vi "Taher.vi"() -> ()   [LabVIEW 2017]
doc: "I. Description:\nThis example demonstrates how to continuously acquire and generate data at the same time, synchronized with one another.\n\nII. Instructions for Running:\n1. Select the physical channel to correspond to where your signal is input on the DAQ device. Also, select the corresponding channel for where your signal is being generated.\n2. Enter the minimum and maximum voltage ranges.\nNote: For better accuracy try to match the input range to the expected voltage level of the measured signal.\n3. Set the sample rate of the acquisition.\nNote: The rate should be at least twice as fast as the maximum frequency component of the signal being acquired. \n6. Select the Rate for the generation\n7. Select what type of signal to generate and the amplitude.\nNote: This example requires two DMA channels to run. If your hardware does not support two DMA channels, you need to set the Data Transfer Mechanism property for the Analog Output Task to use \"Interrupts\". The Data Transfer Mechanism property is located in the DAQmx Channel Property hierarchy at:\n\nDAQmx Channel Property Node>>Analog Output>>General Properties>>Advanced>>Data Transfer and Memory>>Data Transfer Mechanism\n\nRefer to your device documentation to determine how many DMA channels are supported for your hardware.\n\nIII. Block Diagram Steps:\n1. Create an analog input voltage channel. Also, create an analog output voltage channel.\n2. Set the rate for the sample clock. Additionally, define the sample mode to be continuous. Also, set the sample clock rate for the signal generation.\n2a. Call the Get Terminal Name with Device Prefix VI. This will take a Task and a terminal and create a properly formatted device + terminal name to use as the source of the Trigger.\n3. Define the parameters for a Digital Edge Start Trigger. Set the Analog output to trigger off the AI Start Trigger. This is an internal trigger signal.\n4. Use the Basic Function Generator VI to create the signal to be generated.\n5. Call the Start VI to arm the two functions. Make sure the analog output is armed before the analog input. This will ensure both will start at the same time.\n6. Read the waveform data in a loop until the user hits the stop button or an error occurs. The Is Task Done? VI is used to check for errors in the Analog Output Task.\n7. Call the Clear VI to Clear the Task\n8. Use the popup dialog box to display an error if any.\n\nIV. I/O Connections Overview:\nMake sure your signal input/output terminals match the Physical Channel I/O controls."
uses:
  <vilib>/Utility/error.llb/DialogType.ctl
  <vilib>/DAQmx/configure/timing.llb/DAQmx Timing (Sample Clock).vi
  <vilib>/DAQmx/create/channels.llb/DAQmx Create Channel (AI-Voltage-Basic).vi
  <vilib>/DAQmx/create/channels.llb/DAQmx Create Channel (AO-Voltage-Basic).vi
  <vilib>/DAQmx/read.llb/DAQmx Read (Analog 1D DBL NChan 1Samp).vi
  <vilib>/DAQmx/write.llb/DAQmx Write (Analog DBL 1Chan 1Samp).vi
  <vilib>/Utility/file.llb/Write To Spreadsheet File (DBL).vi
  <vilib>/DAQmx/write.llb/DAQmx Write (Analog 2D DBL NChan NSamp).vi
  <vilib>/DAQmx/configure/trigger.llb/DAQmx Start Trigger (Digital Edge).vi
  <vilib>/DAQmx/read.llb/DAQmx Read (Analog DBL 1Chan 1Samp).vi
  pid/pid.llb/PID (DBL).vi
  pid/pid.llb/PID Output Rate Limiter (DBL).vi
  <vilib>/DAQmx/write.llb/DAQmx Write (Analog 1D DBL NChan 1Samp).vi
  <vilib>/ptbypt/NI_PtbyPt.lvlib
  <resource>/objmgr/daqmx.rc
  <vilib>/Analysis/NI_AALBase.lvlib
  <vilib>/Analysis/baseanly.llb/Mean (DBL).vi
  <vilib>/Analysis/NI_AALPro.lvlib
  <vilib>/Utility/file.llb/Write To Spreadsheet File (string).vi
panel:
  in  "Current Amplifier\n1/Gain  (A/V)":dbl=1.0 format="%#_13g"
  out "date/time string":string
  out "Bias Sweep 2":dbl[](graph)
  out "Array":dbl[](array[numeric])
  out "intercept":dbl
  out "Resistance \n[AI1 must be Vout]":dbl
  out "RTD-IV":cluster{dbl[], dbl[]}(graph)
  in  "Bias Offset Correct":dbl
  out "Bias Sweep":dbl[](graph)
  out "element":dbl
  out "mean":dbl format="%.6f"
  out "size(s)":i32
  out "Numeric":i32
  in  "PID":bool=TRUE caption="Step Z"
  in  "Tab Control":enum32{"PID Controller", "Tapping Controls"}(tab)=enum."Tapping Controls"
  in  "Proportional Gain":dbl=0.0001
  in  "Integral Gain":dbl=1e-07
  in  "Differential Gain":dbl=1e-05
  in  "Setpoint":dbl=0.1
  in  "Piezo Delta rate":dbl=1000.0
  in  "Min Current":dbl=0.002
  in  "Max Current":dbl=10.2
  in  "Ramp Rate":dbl=20.0
  in  "Make Contact":i32=1200
  in  "Break Contact":i32=500
  in  "Step Length":i32=100
  in  "Step Max":dbl=0.3
  in  "Step Min":dbl=0.05
  out "Tapping Stop":bool
  out "Case":i32
  in  "Contact Cycles":i32
  in  "Tapping":bool caption="Step Z"
  out "x/y":dbl
  out "Waveform Chart":dbl(graph)
  in  "Analog Ouyput 1":dbl(slide) min=-10.0 max=10.0 step=0.001 scale=-10.0..10.0
  in  "Manual Z":bool caption="Step Z"
  in  "Sweep Amplitude":dbl=1.0
  in  "Stop Sweep":bool
  out "Connections 2":string="AI0=Current\nAI1=Bias\nAI2=dI/dV\nAI3=d2I/dV2\nAI4=X-Axis\nAI5=Z-Axis\n"
  out "Connections":string="AO0=Bias\nAO1=Z-axis\nAO2=X-Axis\nAO3=NA"
  out "Save Indicator":bool
  in  "Z-Direction":bool caption="Step Z"
  in  "Update Bias":bool
  in  "Save IV":bool
  in  "Save Decay":bool
  in  "Sweep Bias":bool
  in  "Step Z":bool
  in  "Comments and Experimental Notes":string="Molecule=TP4\nGain=10nA\nBias Gain=div/1\nSweep Freq.=0.0008Hz\nRef. Bias=4mV\nRef. Freq=2.977kHz\nGain LIA1=2mV\nTC LIA1=1s\nGain LIA2=5mV\nTC LIA2=1s\nLIA1=EGG\nLIA2=SRS\nEGG is driving(possible 5mV offset)"
  in  "Filenumber":i32
  in  "DATA Filename":string="Data_"
  in  "Data Directory":path=path "E:/Research/Data"
  out "Current Decay":cluster{dbl[], dbl[]}(graph)
  out "d2I/dV2":cluster{dbl[], dbl[]}(graph)
  out "dI/dV":cluster{dbl[], dbl[]}(graph)
  out "IV":cluster{dbl[], dbl[]}(graph)
  in  "# Samples":i32=2000
  in  "Frequency (Hz)":dbl=1.0
  out "Measurement 2":cluster{i32, dbl, dbl[]}(graph) caption="Measurement"
  out "Actual Update Generation Rate 2":dbl=5000.0 caption="Actual Update Generation Rate" format="%0.2f"
  in  "stop 3":bool
  in  "Bias":dbl=0.1 caption="Bias Start Point" step=0.1 format="%_3g"
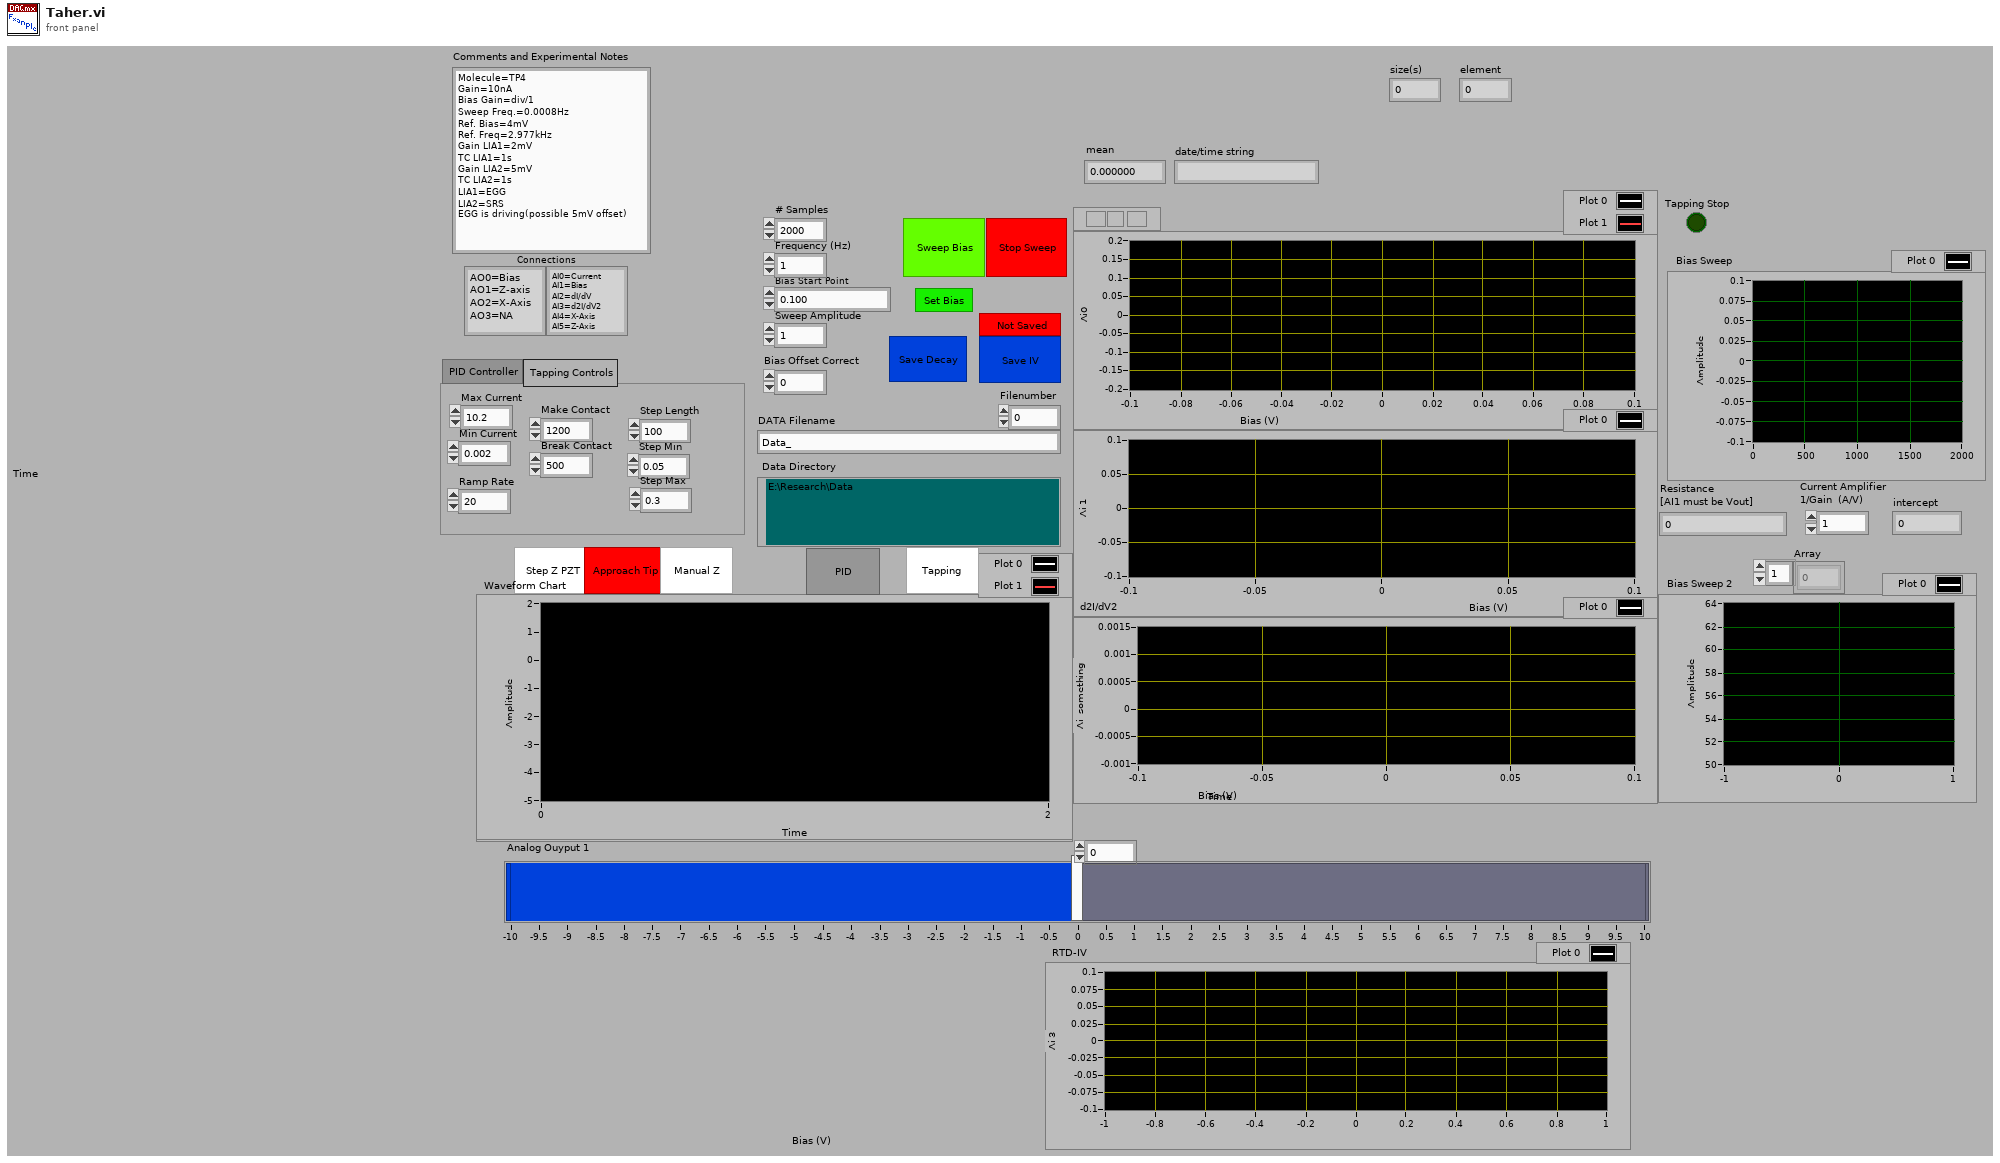
[diagram p1: front panel]
types:
  T1 = enum16{"open", "replace", "create", "open or create", "replace or create", "replace or create with confirmation"}
  T2 = typedef "DialogType.ctl" = u16
  T3 = cluster{"Proportional Gain":dbl, "Integral Gain ":dbl, "Differential Gain":dbl}
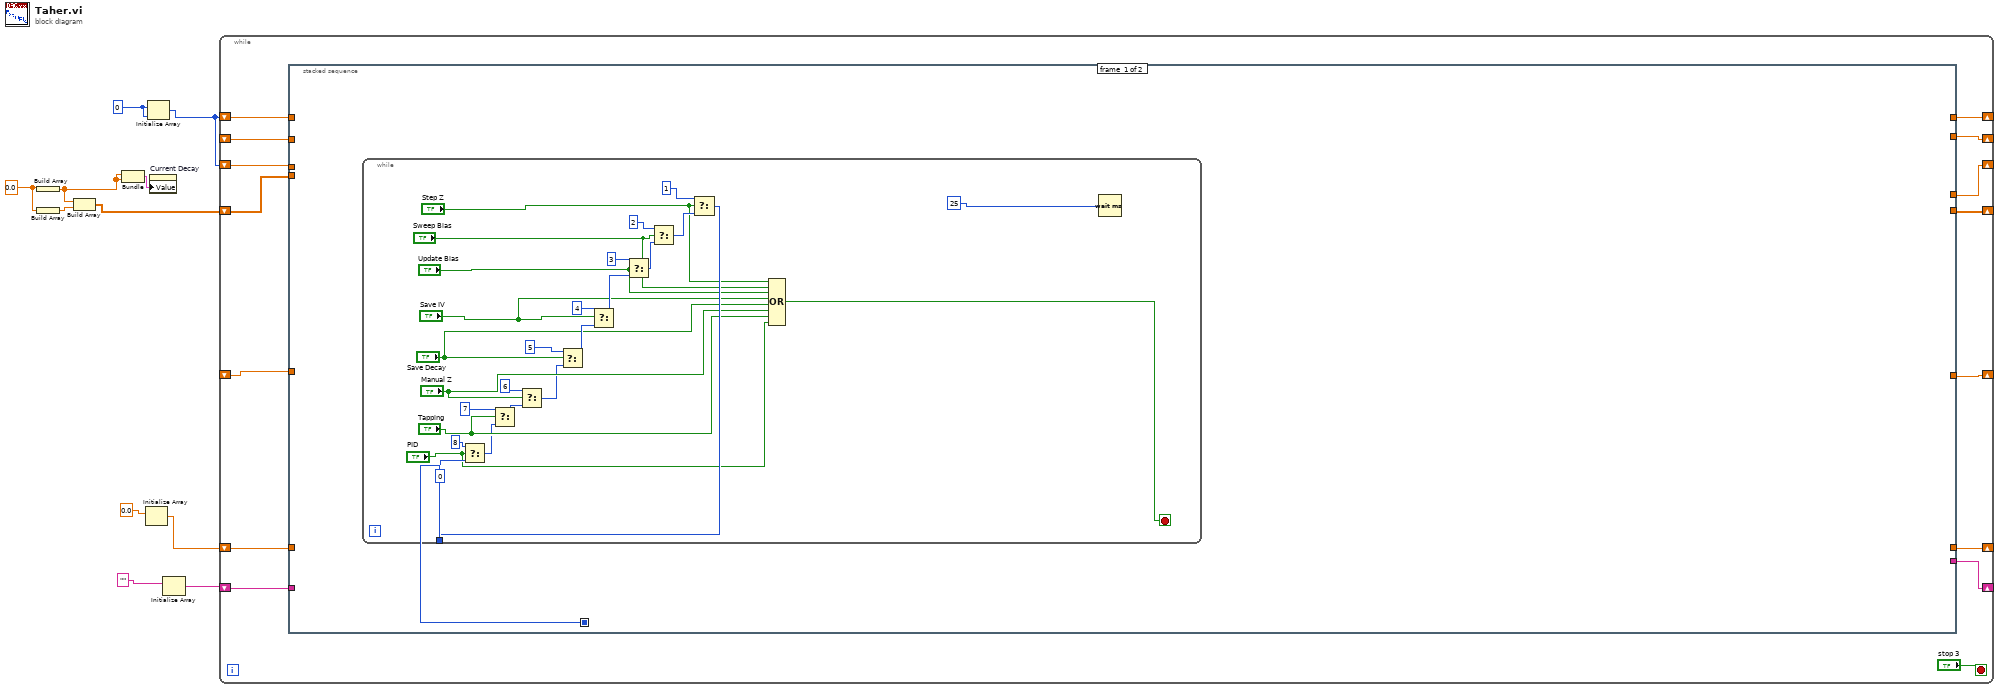
[diagram p0: block diagram]
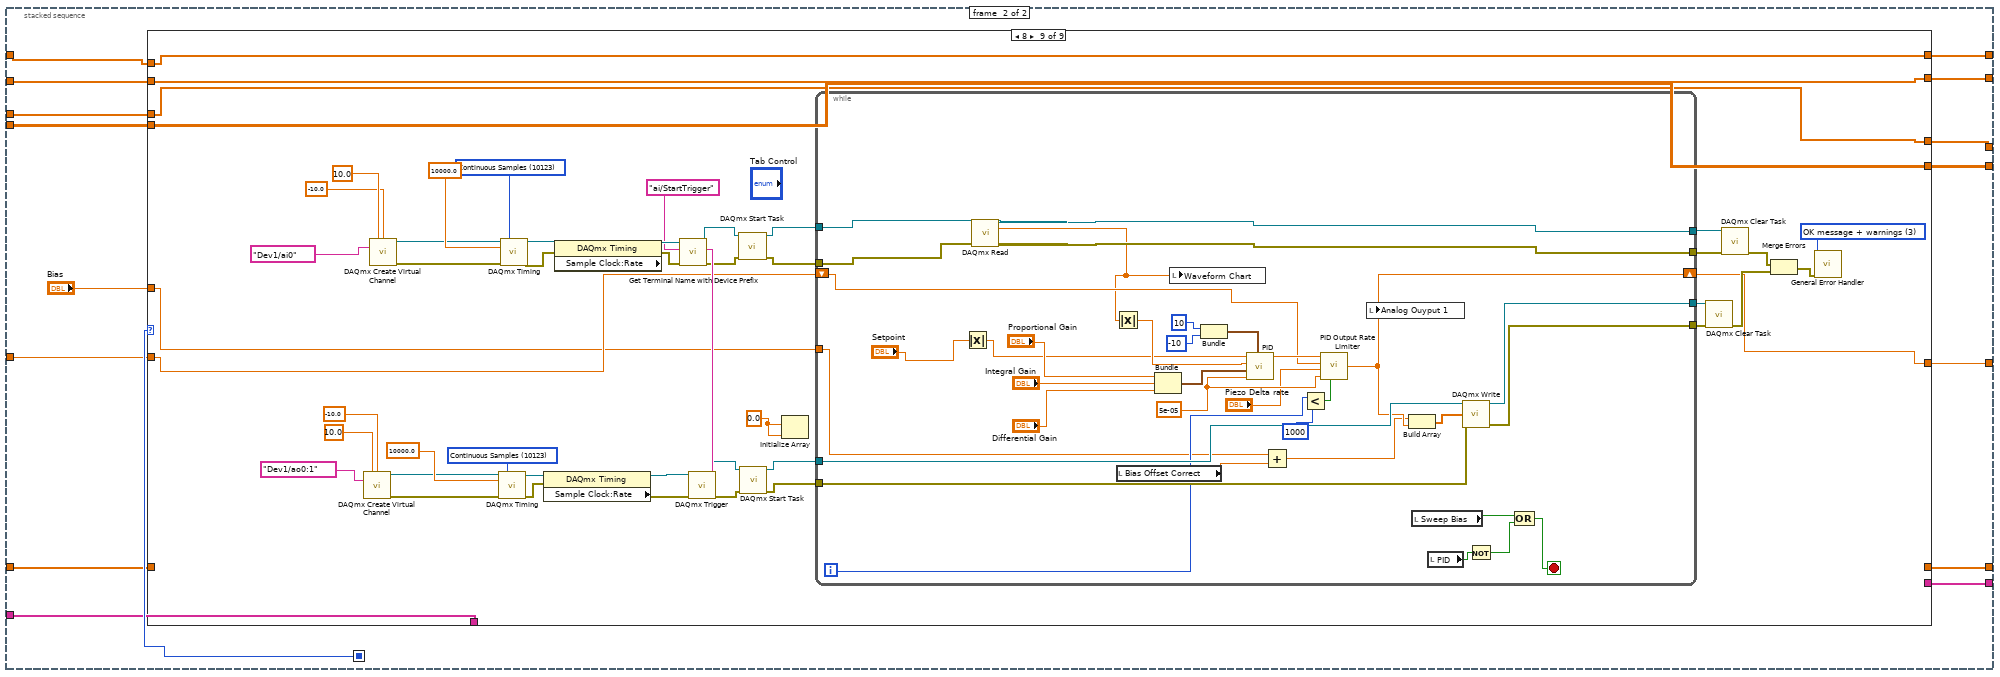
[diagram p2: hidden frame]
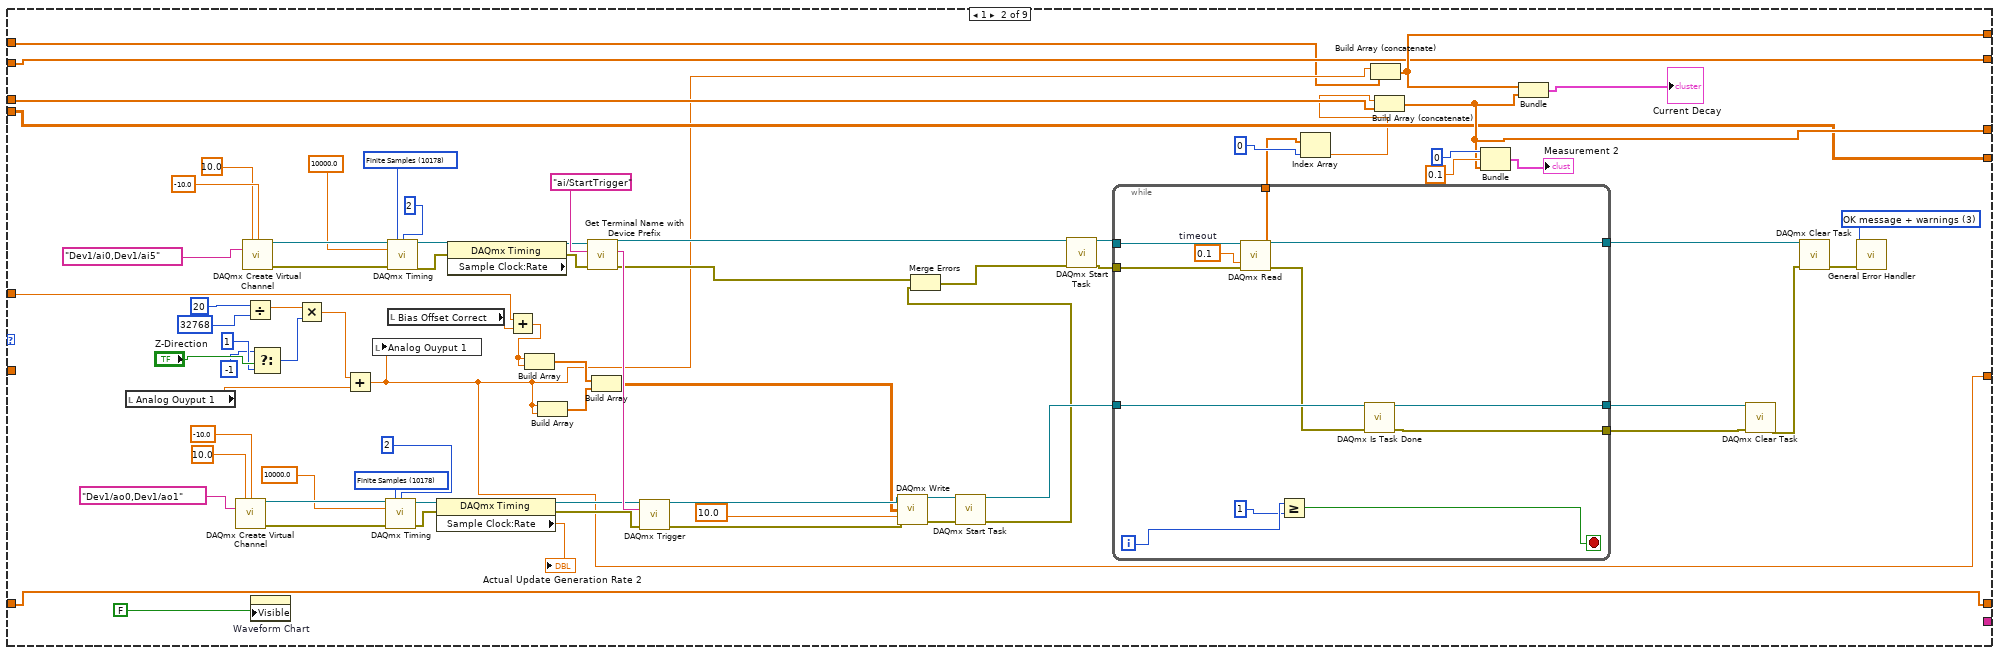
[diagram p4: hidden frame]
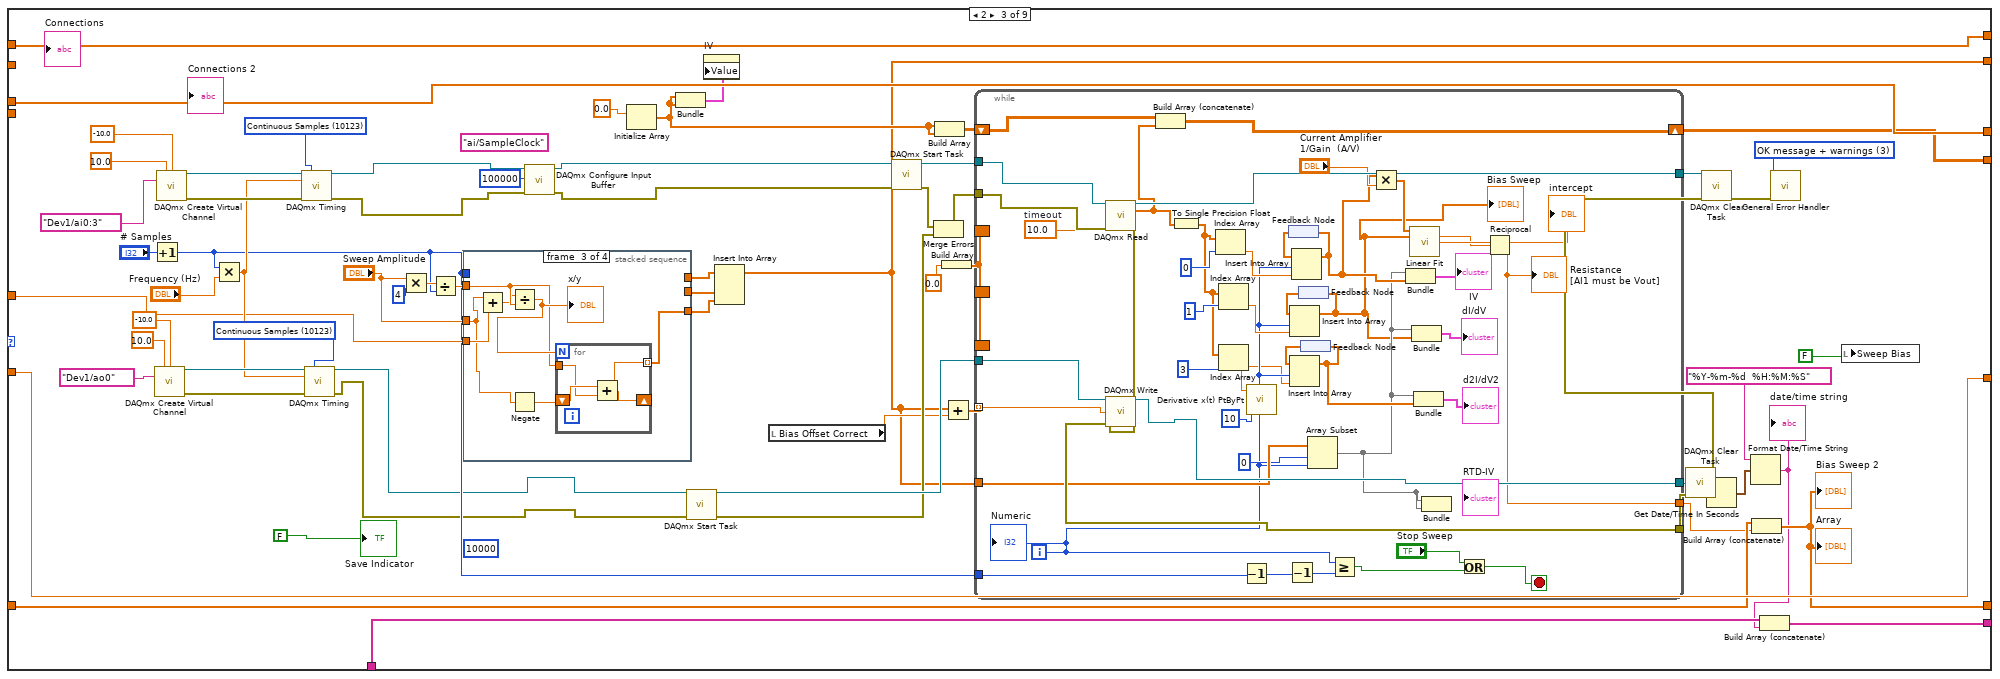
[diagram p5: hidden frame]
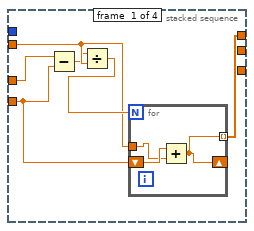
[diagram p6: hidden frame]
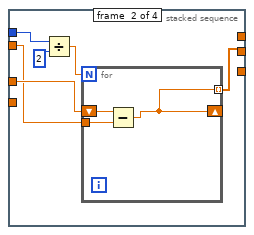
[diagram p7: hidden frame]
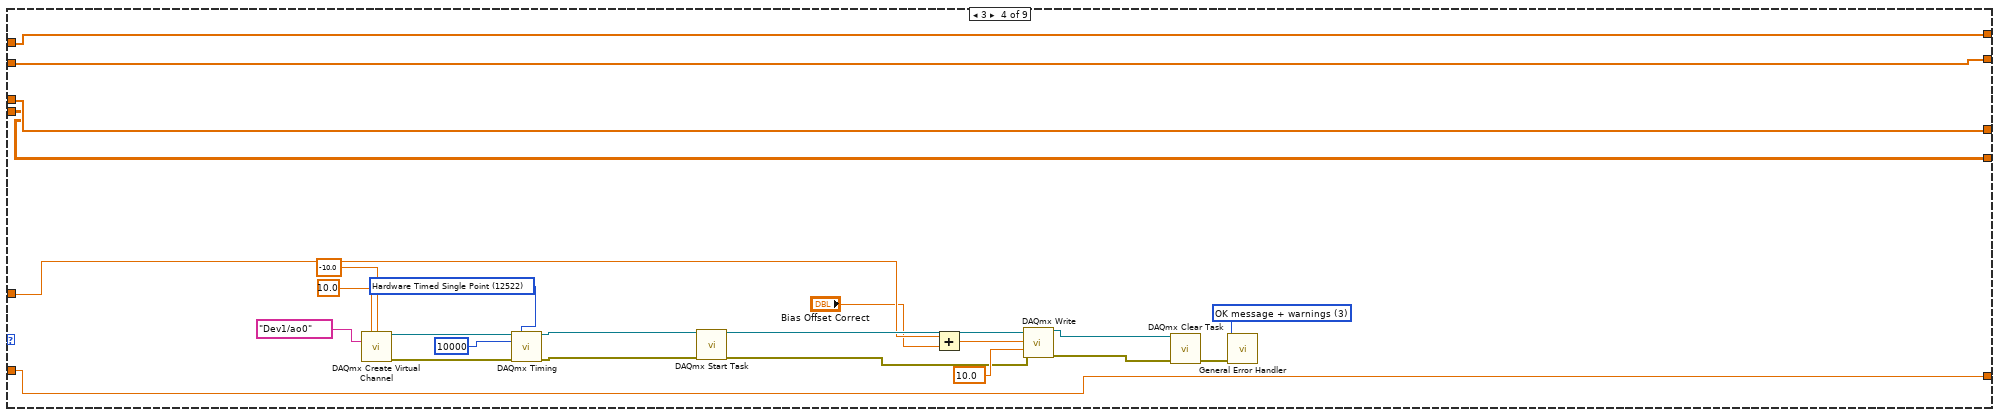
[diagram p9: hidden frame]
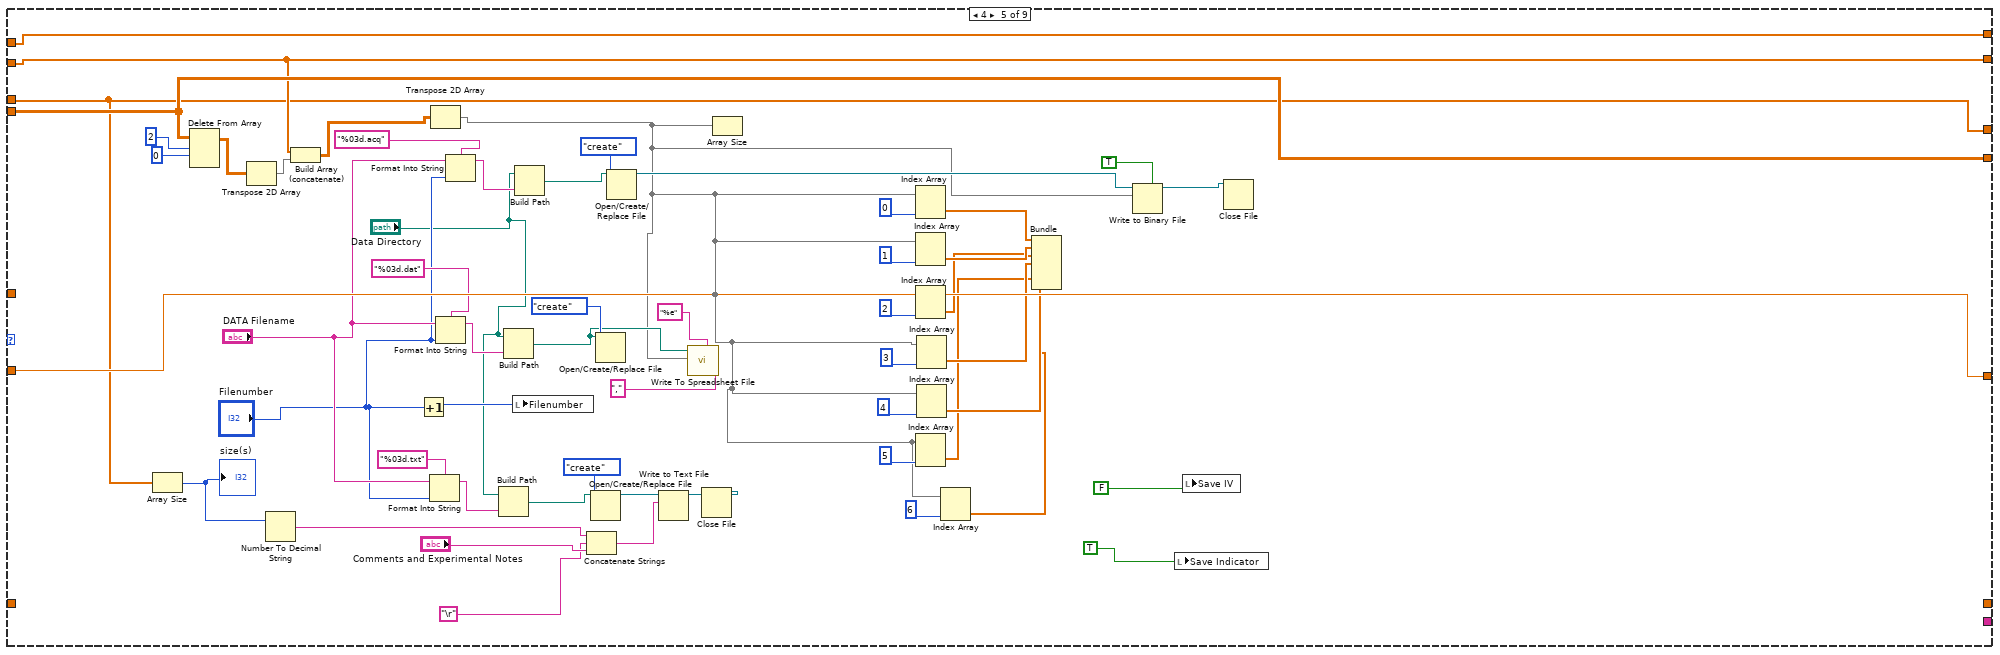
[diagram p10: hidden frame]
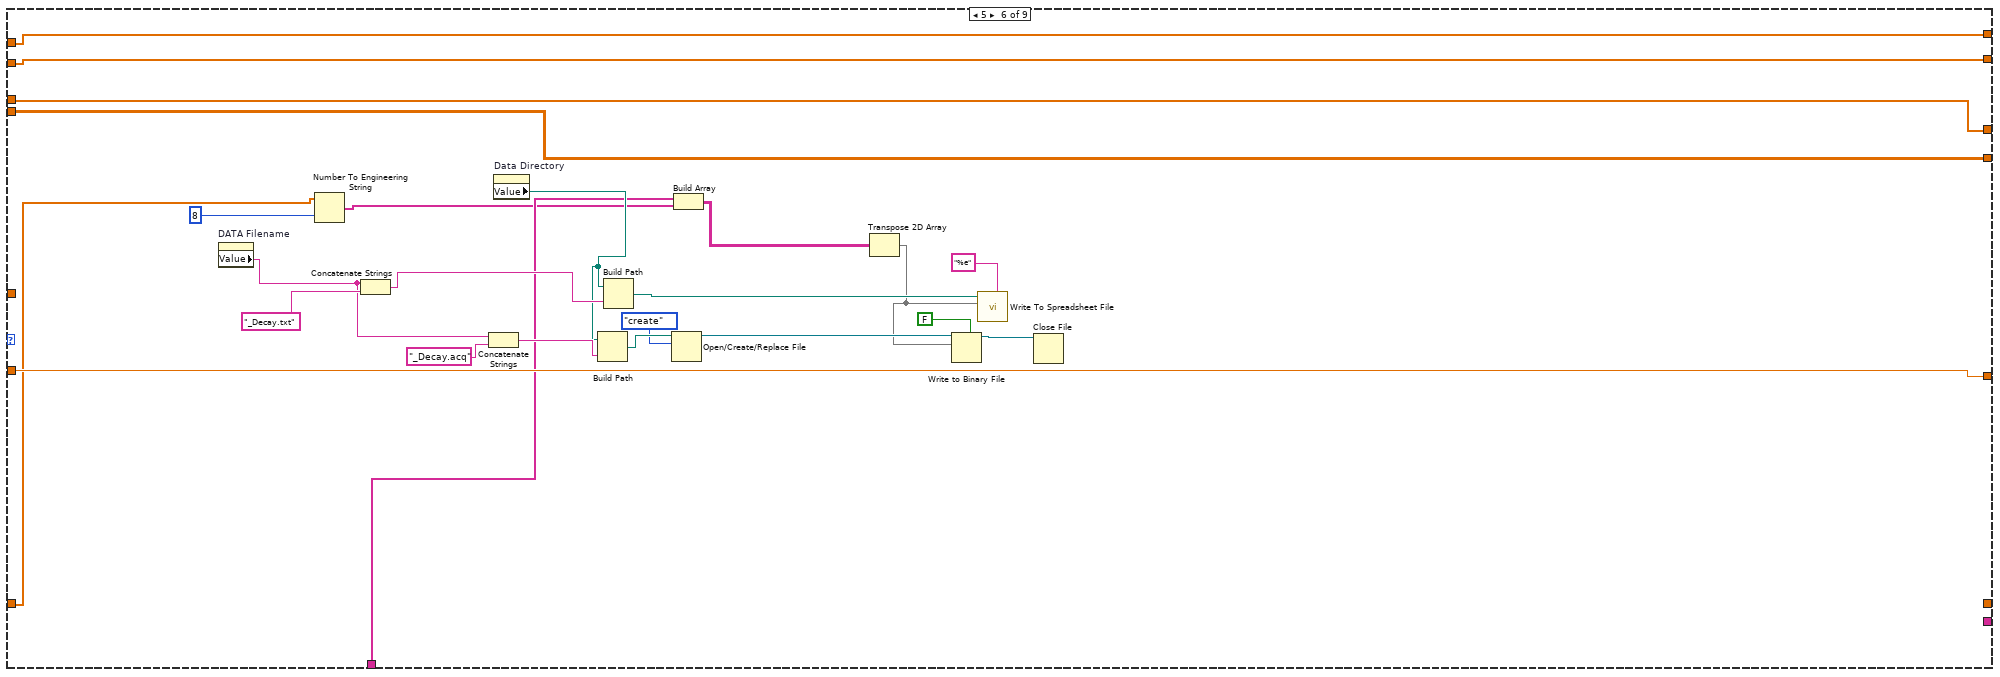
[diagram p11: hidden frame]
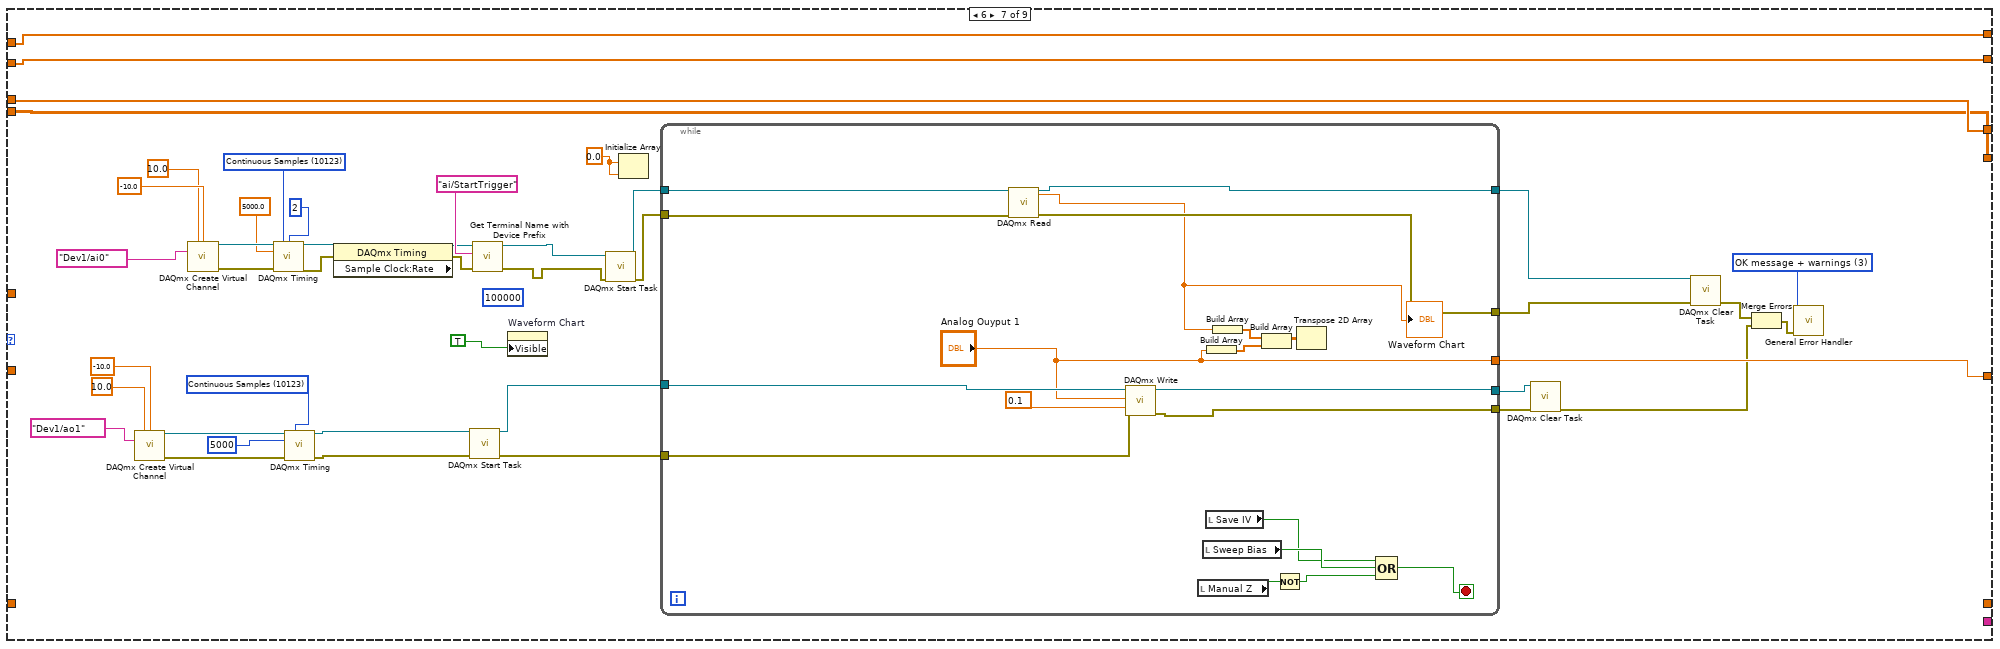
[diagram p12: hidden frame]
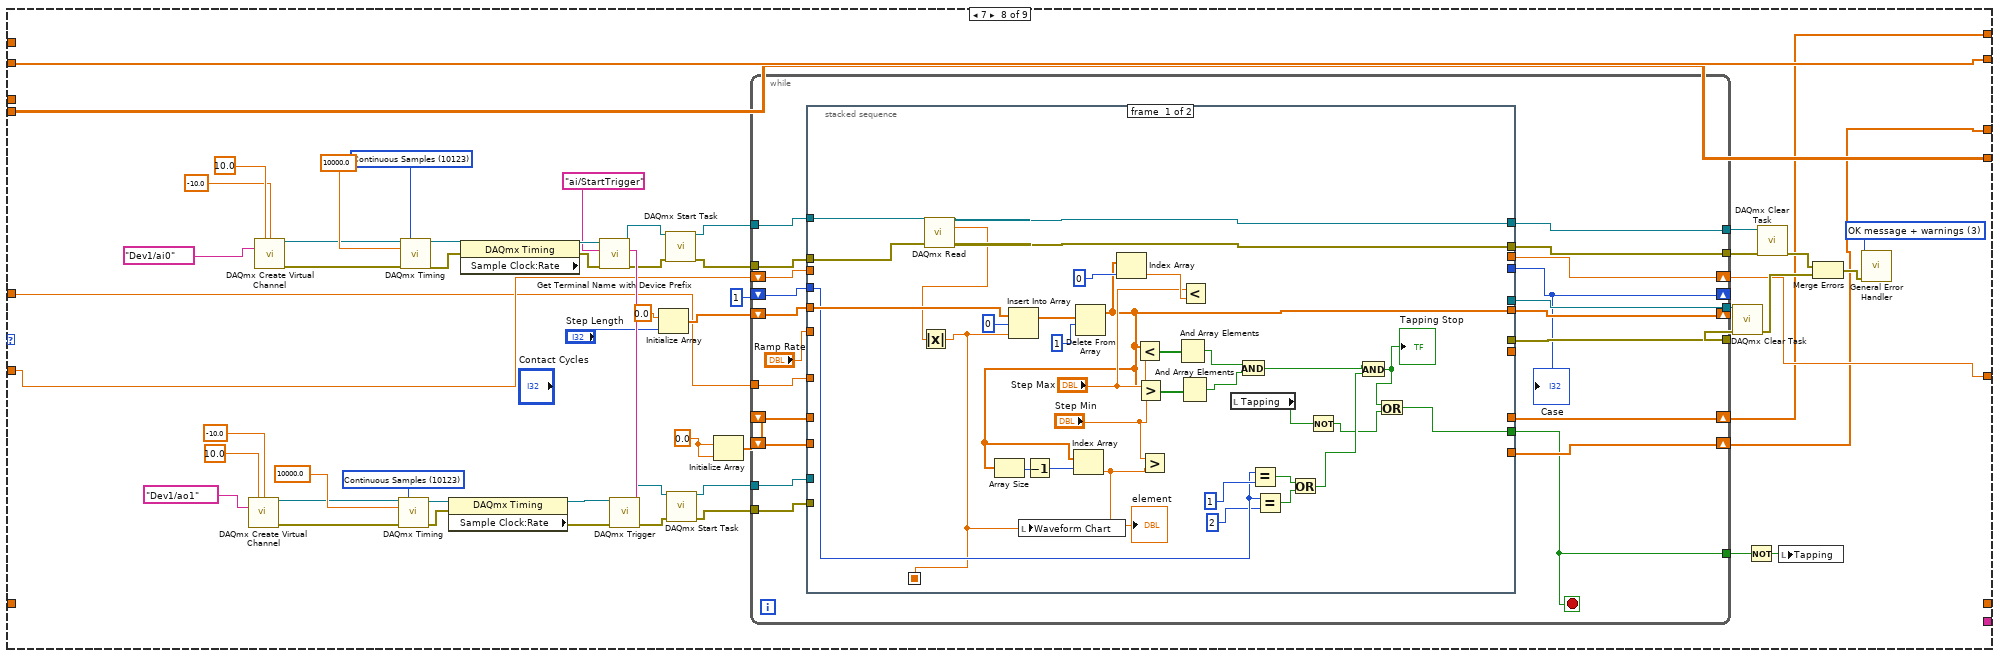
[diagram p13: hidden frame]
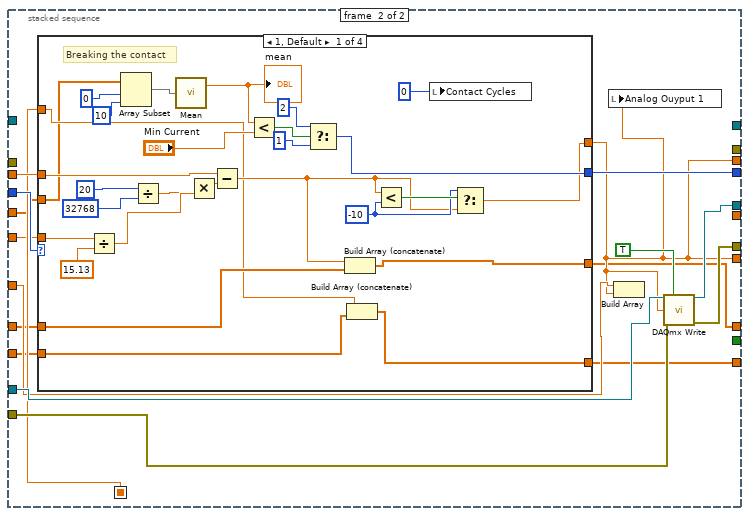
[diagram p14: hidden frame]
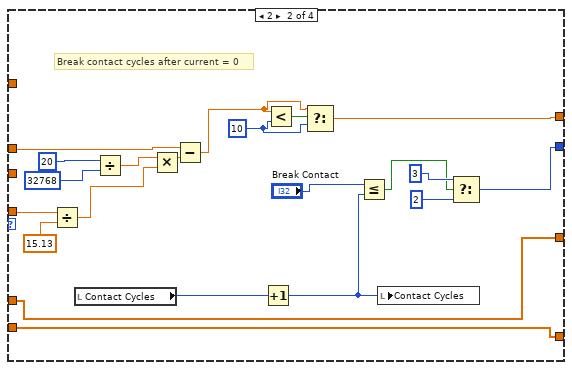
[diagram p15: hidden frame]
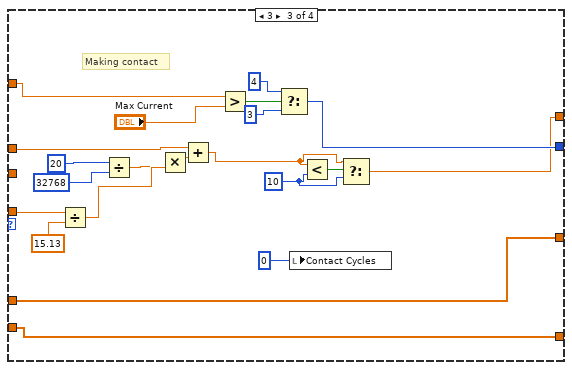
[diagram p16: hidden frame]
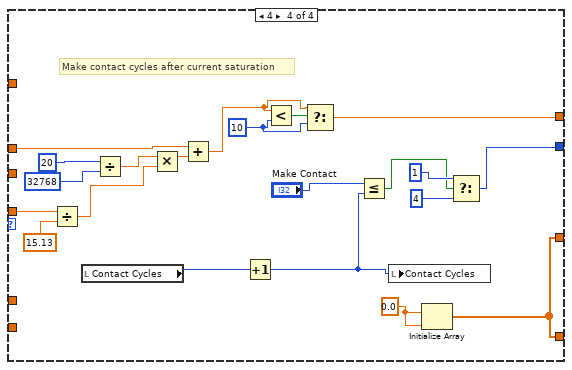
[diagram p17: hidden frame]
diagram:
  w6 = 0
  w11 = 0.0
  n1 = Build Array(w11) -> (w8:dbl[])
  n2 = Build Array(w11) -> (w10:dbl[])
  n3 = Build Array(w8, w10) -> (w9:dbl[][])
  n4 = Bundle(w8, w8) -> (w7:cluster{dbl[], dbl[]})  [unwired: 1 in]
  n5 = Initialize Array(0.0) -> (w3:dbl[])  [unwired: 1 in]
  n6 = Initialize Array(w6, w6) -> (w5:i32[])
  n7 = property on="Current Decay" class="XYGraph (strict)"("Value"=w7) -> ()  [unwired: 2 in, 2 out]
  n8 = Initialize Array("") -> (w1:string[])  [unwired: 1 in]
  n9 = while {
    shift-right: [w24] -> _
    shift-left: w5 -> [w25]
    shift-right: [w22] -> _
    shift-left: w5 -> [w23]
    shift-right: [w20] -> _
    shift-left: _ -> [w21]
    shift-right: [w18] -> _
    shift-left: w9 -> [w19]
    shift-right: [w16] -> _
    shift-left: _ -> [w17]
    shift-right: [w15] -> _
    shift-left: w3 -> [w14]
    shift-right: [w12] -> _
    shift-left: w1 -> [w13]
    stop <- "stop 3" stop-if-true
    n10 = stacked-sequence {
      seq-local: [w27 _] -> [_ w70]
      tunnel: w25 -> [_ w69]
      tunnel: [_ w68] -> w24
      tunnel: w23 -> [_ w66]
      tunnel: [_ w65] -> w22
      tunnel: w21 -> [_ w64]
      tunnel: [_ w59] -> w20
      tunnel: w19 -> [_ w63]
      tunnel: [_ w62] -> w18
      tunnel: w17 -> [_ w61]
      tunnel: [_ w60] -> w16
      tunnel: w14 -> [_ w58]
      tunnel: [_ w57] -> w15
      tunnel: w13 -> [_ w56]
      tunnel: [_ w55] -> w12
      frame #0 {
        n11 = while {
          tunnel: [w45] -> w27
          stop <- w44 stop-if-true
          n12 = Select(t=8, s="PID", f=0) -> (s? t:f=w31:i32)
          n13 = Select(t=7, s="Tapping", f=w31) -> (s? t:f=w33:i32)
          n14 = Select(t=6, s="Manual Z", f=w33) -> (s? t:f=w34:i32)
          n15 = Select(t=5, s="Save Decay", f=w34) -> (s? t:f=w50:i32)
          n16 = Select(t=4, s="Save IV", f=w50) -> (s? t:f=w49:i32)
          n17 = Select(t=3, s="Update Bias", f=w49) -> (s? t:f=w47:i32)
          n18 = Select(t=2, s="Sweep Bias", f=w47) -> (s? t:f=w54:i32)
          n19 = Select(t=1, s="Step Z", f=w54) -> (s? t:f=w45:i32)
          n20 = Compound Arithmetic op=OR("Step Z", "Sweep Bias", "Update Bias", "Save IV", "Save Decay", "Manual Z", "Tapping", "PID") -> (w44:bool)
          n21 = Wait (ms)(milliseconds to wait=25) -> ()  [unwired: 1 out]
        }
      }
      frame #1 {
        n22 = case shown="8" w70 {
          tunnel: w69 -> [w77 w85 w214 w310 w330 w386 w446 _ w686]
          tunnel: [w77 w98 w214 w310 w330 w386 w446 w472 w686] -> w68
          tunnel: "Bias" -> [_ w81 w199 w304 _ _ _ w478 w685]
          tunnel: w66 -> [w76 w82 w211 w311 w377 w402 w448 _ w687]
          tunnel: [w76 w99 w211 w311 w377 w402 w448 w473 w687] -> w65
          tunnel: w64 -> [w75 _ w210 w309 w376 w403 _ w479 w694]
          tunnel: [w75 w83 w210 w309 w376 w403 w417 w474 w691] -> w59
          tunnel: w63 -> [w74 w96 _ w307 w356 w404 w445 w476 w692]
          tunnel: [w74 w96 w191 w307 w356 w404 w445 w476 w692] -> w62
          tunnel: [w73 w91 w174 w306 w354 w387 w447 w477 w693] -> w60
          tunnel: w61 -> [w73 w91 _ w306 w354 w387 w447 w477 w693]
          tunnel: w58 -> [w72 w78 w173 _ _ w384 _ _ _]
          tunnel: [w72 w78 w171 _ _ _ _ _ _] -> w57
          tunnel: w56 -> [w71 _ w170 _ _ w385 _ _ _]
          tunnel: [w71 _ w169 _ _ _ _ _ _] -> w55
          frame 0, Default {
          }
          frame 1 {
            w133 = T2 3 items=["no dialog", "OK message", "continue or stop message", "OK message + warnings", "continue/stop + warnings"] ("type of dialog (OK msg:1)")
            w145 = 10178 items=["Finite Samples"=10178, "Continuous Samples"=10123] ("sample mode")
            w150 = 10178 items=["Finite Samples"=10178, "Continuous Samples"=10123] ("sample mode")
            n23 = local read "Analog Ouyput 1"() -> (w86:dbl)
            n24 = call-poly <vilib>:"DAQmx Create Virtual Channel.vi"("maximum value"=10.0 ("maximum value 2"), "minimum value"=-10.0 ("minimum value 2"), "physical channels"=tag "Dev1/ao0,Dev1/ao1" ("physical channels 2")) -> ("task out"=w144:refnum<k21>, "error out"=w143:errorcluster)  [unwired: 11 in]
            n25 = call-poly <vilib>:"DAQmx Create Virtual Channel.vi"("maximum value"=10.0 ("Maximum Value 2"), "minimum value"=-10.0 ("Minimum Value 2"), "physical channels"=tag "Dev1/ai0,Dev1/ai5" ("Physical Channel 2")) -> ("task out"=w148:refnum<k21>, "error out"=w149:errorcluster)  [unwired: 11 in]
            n26 = Divide(x=20, y=32768) -> (x/y=w95:dbl)
            n27 = property on="Waveform Chart" class="WFChart (strict)"("Visible"=FALSE) -> ()  [unwired: 2 in, 2 out]
            n28 = Select(t=-1 ("f"), s="Z-Direction", f=1) -> (s? t:f=w93:i32)
            n29 = Multiply(x=w95, y=w93) -> (x*y=w94:dbl)
            n30 = Add(x=w94, y=w86) -> (x+y=w83:dbl)
            n31 = local write "Analog Ouyput 1"(w83) -> ()
            n32 = call-poly <vilib>:"DAQmx Timing.vi"("task/channels in"=w144, "sample mode"=w145, "samples per channel"=2, "rate"=10000.0 ("rate 2"), "error in"=w143) -> ("task out"=w128:refnum<k21>, "error out"=w127:errorcluster)  [unwired: 9 in]
            n33 = call-poly <vilib>:"DAQmx Timing.vi"("task/channels in"=w148, "sample mode"=w150, "samples per channel"=2, "rate"=10000.0 ("Rate 2"), "error in"=w149) -> ("task out"=w122:refnum<k21>, "error out"=w121:errorcluster)  [unwired: 9 in]
            n34 = local read "Bias Offset Correct"() -> (w80:dbl)
            n35 = property class="DAQmx Timing"(reference=w128, error in=w127) -> (reference out=w129:refnum<k21>, error out=w126:errorcluster, "Sample Clock:Rate"=→"Actual Update Generation Rate 2":dbl)
            n36 = property class="DAQmx Timing" props=["Sample Clock:Rate"](reference=w122, error in=w121) -> (reference out=w120:refnum<k21>, error out=w119:errorcluster)  [unwired: 1 out]
            n37 = Add(x=w81, y=w80) -> (x+y=w79:dbl)
            n38 = Build Array(w79, w79) -> (w106:dbl[])
            n39 = Build Array(w83, w83) -> (w105:dbl[])
            n40 = call "Get Terminal Name with Device Prefix.vi"("error in (no error)"=w119, "Local Terminal Name"="ai/StartTrigger" ("terminal"), "task/channels in"=w120) -> ("error out"=w125:errorcluster, "Terminal Name with Device Prefix"=w130:tag, "task out"=w110:refnum<k21>)  [unwired: 6 in]
            n41 = Build Array(w106, w105) -> (w104:dbl[][])
            n42 = call-poly <vilib>:"DAQmx Trigger.vi"("task/channels in"=w129, "source"=w130, "error in"=w126) -> ("task out"=w135:refnum<k21>, "error out"=w136:errorcluster)  [unwired: 11 in]
            n43 = call-poly <vilib>:"DAQmx Write.vi"("task/channels in"=w135, "data"=w104, "timeout"=10.0 ("Wirite Timeout"), "error in"=w136) -> ("task out"=w138:refnum<k21>, "error out"=w137:errorcluster)  [unwired: 9 in, 1 out]
            n44 = call <vilib>:"DAQmx Start Task.vi"("task/channels in"=w138, "error in"=w137) -> ("task out"=w142:refnum<k21>, "error out"=w124:errorcluster)  [unwired: 12 in]
            n45 = Merge Errors(w125, w124) -> (w112:errorcluster)
            n46 = call <vilib>:"DAQmx Start Task.vi"("task/channels in"=w110, "error in"=w112) -> ("task out"=w109:refnum<k21>, "error out"=w111:errorcluster)  [unwired: 12 in]
            n47 = while {
              tunnel: [w165] -> w151
              tunnel: w142 -> [w164]
              tunnel: [w163] -> w141
              tunnel: w109 -> [w154]
              tunnel: [w162] -> w118
              tunnel: [w159] -> w102
              tunnel: w111 -> [w155]
              i -> [w158]
              stop <- w156 stop-if-true
              w161 = 0.1  # timeout
              n48 = call-poly <vilib>:"DAQmx Read.vi"("task/channels in"=w154, "timeout"=w161, "error in"=w155) -> ("task out"=w165:refnum<k21>, "data"=w159:dbl[], "error out"=w160:errorcluster)  [unwired: 10 in]
              n49 = Greater Or Equal?(x=w158, y=1) -> (x >= y?=w156:bool)
              n50 = call <vilib>:"DAQmx Is Task Done.vi"("task/channels in"=w164, "error in"=w160) -> ("task out"=w163:refnum<k21>, "error out"=w162:errorcluster)  [unwired: 11 in, 1 out]
            }
            n51 = Index Array(array=w102, index=0) -> (element=w84:dbl)
            n52 = Build Array (concatenate)(w83, w82) -> (w99:dbl[])
            n53 = Build Array (concatenate)(w84, w85) -> (w98:dbl[])
            n54 = Bundle(0, 0.1, w98) -> (→"Measurement 2":cluster{i32, dbl, dbl[]})  [unwired: 1 in]
            n55 = Bundle(w99, w98) -> (→"Current Decay":cluster{dbl[], dbl[]})  [unwired: 1 in]
            n56 = call <vilib>:"DAQmx Clear Task.vi"("task in"=w141, "error in"=w118) -> ("error out"=w117:errorcluster)  [unwired: 13 in]
            n57 = call <vilib>:"DAQmx Clear Task.vi"("task in"=w151, "error in"=w117) -> ("error out"=w116:errorcluster)  [unwired: 13 in]
            n58 = call <vilib>:"General Error Handler.vi"("type of dialog (OK msg:1)"=w133, "error in (no error)"=w116) -> ()  [unwired: 9 in, 5 out]
          }
          frame 2 {
            (unwired) 10000
            w208 = 10123 items=["Finite Samples"=10178, "Continuous Samples"=10123, "Hardware Timed Single Point"=12522] ("sample mode")
            w209 = 10123 items=["Finite Samples"=10178, "Continuous Samples"=10123, "Hardware Timed Single Point"=12522] ("sample mode")
            (unwired) "ai/SampleClock" ("terminal")
            w219 = T2 3 items=["no dialog", "OK message", "continue or stop message", "OK message + warnings", "continue/stop + warnings"] ("type of dialog (OK msg:1)")
            n59 = Increment(x="# Samples") -> (x+1=w189:i32)
            n60 = call-poly <vilib>:"DAQmx Create Virtual Channel.vi"("maximum value"=10.0, "minimum value"=-10.0, "physical channels"=tag "Dev1/ao0") -> ("task out"=w222:refnum<k21>, "error out"=w221:errorcluster)  [unwired: 11 in]
            n61 = call-poly <vilib>:"DAQmx Create Virtual Channel.vi"("maximum value"=10.0 ("Maximum Value"), "minimum value"=-10.0 ("Minimum Value"), "physical channels"=tag "Dev1/ai0:3" ("Physical Channel")) -> ("task out"=w226:refnum<k21>, "error out"=w227:errorcluster)  [unwired: 11 in]
            n62 = Multiply(x=w189, y="Frequency (Hz)") -> (x*y=w213:dbl)
            n63 = call-poly <vilib>:"DAQmx Timing.vi"("task/channels in"=w226, "sample mode"=w208, "rate"=w213, "error in"=w227) -> ("task out"=w183:refnum<k21>, "error out"=w181:errorcluster)  [unwired: 10 in]
            n64 = call-poly <vilib>:"DAQmx Timing.vi"("task/channels in"=w222, "sample mode"=w209, "rate"=w213, "error in"=w221) -> ("task out"=w178:refnum<k21>, "error out"=w177:errorcluster)  [unwired: 10 in]
            n65 = Multiply(x="Sweep Amplitude", y=4) -> (x*y=w197:dbl)
            n66 = Divide(x=w197, y=w189) -> (x/y=w196:dbl)
            n67 = stacked-sequence {
              tunnel: "Sweep Amplitude" -> [w280 w286 w294 _]
              tunnel: w199 -> [w278 _ w298 _]
              tunnel: w196 -> [w276 w285 w296 _]
              tunnel: [w277 _ _ _] -> w195
              tunnel: w189 -> [_ w289 _ _]
              tunnel: [_ w284 _ _] -> w194
              tunnel: [_ _ w297 _] -> w193
              frame #0 {
                n68 = Subtract(x=w280, y=w278) -> (x-y=w275:dbl)
                n69 = Divide(x=w275, y=w276) -> (x/y=w279:dbl)
                n70 = for {
                  N: w279 -> [_]
                  tunnel: w276 -> [w282]
                  shift-right: [w281] -> _
                  shift-left: w278 -> [w283]
                  tunnel: [w281] -> w277 mode=indexing
                  n71 = Add(x=w283, y=w282) -> (x+y=w281:dbl)
                }
              }
              frame #1 {
                n72 = Divide(x=w289, y=2) -> (x/y=w287:dbl)
                n73 = for {
                  N: w287 -> [_]
                  tunnel: w285 -> [w291]
                  shift-right: [w290] -> _
                  shift-left: w286 -> [w292]
                  tunnel: [w290] -> w284 mode=indexing
                  n74 = Subtract(x=w292, y=w291) -> (x-y=w290:dbl)
                }
              }
              frame #2 {
                n75 = Add(x=w294, y=w298) -> (x+y=w295:dbl)
                n76 = Divide(x=w295, y=w296) -> (x/y=w299:dbl)
                "x/y" <- w299
                n77 = Negate(x=w294) -> (-x=w293:dbl)
                n78 = for {
                  N: w299 -> [_]
                  tunnel: w296 -> [w301]
                  shift-right: [w300] -> _
                  shift-left: w293 -> [w302]
                  tunnel: [w300] -> w297 mode=indexing
                  n79 = Add(x=w302, y=w301) -> (x+y=w300:dbl)
                }
              }
              frame #3 {
              }
            }
            n80 = call <vilib>:"DAQmx Configure Input Buffer.vi"("task/channels in"=w183, "buffer size (in samples per channel)"=100000, "error in"=w181) -> ("task out"=w182:refnum<k21>, "error out"=w180:errorcluster)  [unwired: 11 in]
            n81 = Initialize Array(0.0) -> (w188:dbl[])  [unwired: 1 in]
            n82 = Bundle(w188, w188) -> (w187:cluster{dbl[], dbl[]})  [unwired: 1 in]
            n83 = call <vilib>:"DAQmx Start Task.vi"("task/channels in"=w178, "error in"=w177) -> ("task out"=w207:refnum<k21>, "error out"=w203:errorcluster)  [unwired: 12 in]
            n84 = property on="IV" class="XYGraph (strict)"("Value"=w187) -> ()  [unwired: 2 in, 2 out]
            n85 = Insert Into Array(array=w195, new element #1=w194, new element #2=w193) -> (w174:dbl[])  [unwired: 1 in]
            n86 = local read "Bias Offset Correct"() -> (w175:dbl)
            n87 = call <vilib>:"DAQmx Start Task.vi"("task/channels in"=w182, "error in"=w180) -> ("task out"=w205:refnum<k21>, "error out"=w204:errorcluster)  [unwired: 12 in]
            n88 = Merge Errors(w204, w203) -> (w206:errorcluster)
            n89 = Build Array(w188, w188) -> (w190:dbl[][])
            n90 = Build Array(0.0) -> (w185:dbl[])
            n91 = Add(x=w174, y=w175) -> (x+y=w176:dbl[])
            n92 = while {
              tunnel: [w266] -> w228
              tunnel: [w269] -> w220
              tunnel: [w268] -> w217
              tunnel: w189 -> [w244]
              tunnel: w176 -> [w249] mode=indexing
              tunnel: w207 -> [w271]
              tunnel: w205 -> [w274]
              tunnel: w206 -> [w273]
              shift-right: [w250] -> w191
              shift-left: w190 -> [w267]
              tunnel: w174 -> [w264]
              border: w185 -> [_]
              border: w185 -> [_]
              border: w185 -> [_]
              tunnel: [w236] -> w172
              i -> [w245]
              stop <- w246 stop-if-true
              w270 = 10.0  # timeout
              n93 = call-poly <vilib>:"DAQmx Read.vi"("task/channels in"=w274, "timeout"=w270, "error in"=w273) -> ("task out"=w266:refnum<k21>, "data"=w252:dbl[], "error out"=w272:errorcluster)  [unwired: 10 in]
              n94 = call-poly <vilib>:"DAQmx Write.vi"("task/channels in"=w271, "data"=w249, "error in"=w272) -> ("task out"=w269:refnum<k21>, "error out"=w268:errorcluster)  [unwired: 10 in, 1 out]
              n95 = Build Array (concatenate)(w267, w252) -> (w250:dbl[][])
              n96 = To Single Precision Float(number=w252) -> (single precision float=w251:sgl[])
              n97 = Index Array(array=w251, index=0) -> (element=w262:sgl)
              n98 = Index Array(array=w251, index=1) -> (element=w258:sgl)
              n99 = Index Array(array=w251, index=3) -> (element=w240:sgl)
              n100 = Decrement(x=w244) -> (x-1=w242:i32)
              n101 = call <vilib>:"Derivative x(t) PtByPt.vi"("dt"=10, "x"=w240) -> ()  [unwired: 2 in, 2 out]
              n102 = Decrement(x=w242) -> (x-1=w243:i32)
              n103 = feedback #1() -> (w261:dbl[])
              n104 = Insert Into Array(array=w261, index=w245, new element=w262) -> (w234:dbl[])
              n105 = feedback-in #1(w234) -> ()
              n106 = feedback #2() -> (w257:dbl[])
              n107 = Insert Into Array(array=w257, index=w245, new element=w258) -> (w231:dbl[])
              "Bias Sweep" <- w231
              n108 = feedback-in #2(w231) -> ()
              n109 = feedback #3() -> (w256:dbl[])
              n110 = Insert Into Array(array=w256, index=w245, new element=w240) -> (w239:dbl[])
              n111 = feedback-in #3(w239) -> ()
              n112 = Array Subset(array=w264, index=0, length=w245) -> (w232:dbl[])
              n113 = Greater Or Equal?(x=w245, y=w243) -> (x >= y?=w247:bool)
              n114 = Multiply(x=w234, y="Current Amplifier\n1/Gain  (A/V)") -> (x*y=w233:dbl[])
              n115 = Bundle(w232, w234) -> (→"IV":cluster{dbl[], dbl[]})  [unwired: 1 in]
              n116 = call <vilib>:"Linear Fit.vi"("Y"=w233, "X"=w231) -> ("slope"=w237:dbl, "intercept"=→"intercept":dbl)  [unwired: 9 in, 3 out]
              n117 = Bundle(w232, w231) -> (→"dI/dV":cluster{dbl[], dbl[]})  [unwired: 1 in]
              n118 = Bundle(w232, w239) -> (→"d2I/dV2":cluster{dbl[], dbl[]})  [unwired: 1 in]
              n119 = Bundle(w232, w232) -> ()  [unwired: 1 in, 1 out]
              n120 = Or(x="Stop Sweep", y=w247) -> (x .or. y?=w246:bool)
              n121 = Reciprocal(x=w237) -> (1/x=w236:dbl)
              "Resistance \n[AI1 must be Vout]" <- w236
              "Numeric" <- w245
            }
            n122 = call <vilib>:"DAQmx Clear Task.vi"("task in"=w220, "error in"=w217) -> ("error out"=w216:errorcluster)  [unwired: 13 in]
            n123 = call <vilib>:"DAQmx Clear Task.vi"("task in"=w228, "error in"=w216) -> ("error out"=w215:errorcluster)  [unwired: 13 in]
            n124 = Get Date/Time In Seconds() -> (seconds since 1Jan1904=w167:timestamp)
            n125 = Format Date/Time String(time format string (%c)="%Y-%m-%d  %H:%M:%S", seconds (now)=w167) -> (date/time string=w166:string)  [unwired: 1 in]
            "date/time string" <- w166
            n126 = Build Array (concatenate)(w173, w172) -> (w171:dbl[])
            "Array" <- w171
            "Bias Sweep 2" <- w171
            n127 = Build Array (concatenate)(w170, w166) -> (w169:string[])
            n128 = call <vilib>:"General Error Handler.vi"("type of dialog (OK msg:1)"=w219, "error in (no error)"=w215) -> ()  [unwired: 9 in, 5 out]
            n129 = local write "Sweep Bias"(FALSE) -> ()
            "Save Indicator" <- FALSE
          }
          frame 3 {
            w315 = T2 3 items=["no dialog", "OK message", "continue or stop message", "OK message + warnings", "continue/stop + warnings"] ("type of dialog (OK msg:1)")
            w320 = 12522 items=["Finite Samples"=10178, "Continuous Samples"=10123, "Hardware Timed Single Point"=12522] ("sample mode")
            n130 = call-poly <vilib>:"DAQmx Create Virtual Channel.vi"("maximum value"=10.0 ("maximum value 2"), "minimum value"=-10.0 ("minimum value 2"), "physical channels"=tag "Dev1/ao0" ("physical channels 2")) -> ("task out"=w323:refnum<k21>, "error out"=w322:errorcluster)  [unwired: 11 in]
            n131 = call-poly <vilib>:"DAQmx Timing.vi"("task/channels in"=w323, "sample mode"=w320, "rate"=10000, "error in"=w322) -> ("task out"=w319:refnum<k21>, "error out"=w318:errorcluster)  [unwired: 10 in]
            n132 = call <vilib>:"DAQmx Start Task.vi"("task/channels in"=w319, "error in"=w318) -> ("task out"=w317:refnum<k21>, "error out"=w316:errorcluster)  [unwired: 12 in]
            n133 = Add(x=w304, y="Bias Offset Correct") -> (x+y=w305:dbl)
            n134 = call-poly <vilib>:"DAQmx Write.vi"("task/channels in"=w317, "data"=w305, "timeout"=10.0 ("Wirite Timeout"), "error in"=w316) -> ("task out"=w313:refnum<k21>, "error out"=w312:errorcluster)  [unwired: 9 in, 1 out]
            n135 = call <vilib>:"DAQmx Clear Task.vi"("task in"=w313, "error in"=w312) -> ("error out"=w314:errorcluster)  [unwired: 13 in]
            n136 = call <vilib>:"General Error Handler.vi"("type of dialog (OK msg:1)"=w315, "error in (no error)"=w314) -> ()  [unwired: 9 in, 5 out]
          }
          frame 4 {
            n137 = Array Size(array=w330) -> (size(s)=w329:i32)
            "size(s)" <- w329
            n138 = Delete From Array(array=w356, length=2, index (row)=0) -> (array with subset deleted=w353:dbl[][])  [unwired: 1 in, 1 out]
            n139 = Transpose 2D Array(2D array=w353) -> (transposed array=w352:dbl[][])
            n140 = Number To Decimal String(number=w329) -> (decimal integer string=w328:string)  [unwired: 1 in]
            n141 = Build Array (concatenate)(w354, w352) -> (w334:dbl[][])
            n142 = Increment(x="Filenumber") -> (x+1=w379:i32)
            n143 = Format Into String(format string="%03d.txt", initial string="DATA Filename", "Filenumber") -> (resulting string=w367:string)  [unwired: 1 in, 1 out]
            n144 = Transpose 2D Array(2D array=w334) -> (transposed array=w333:dbl[][])
            n145 = Format Into String(format string="%03d.dat", initial string="DATA Filename", "Filenumber") -> (resulting string=w381:string)  [unwired: 1 in, 1 out]
            n146 = Format Into String(format string="%03d.acq", initial string="DATA Filename", "Filenumber") -> (resulting string=w374:string)  [unwired: 1 in, 1 out]
            n147 = Build Path(base path="Data Directory", name or relative path=w367) -> (appended path=w365:path)
            n148 = Build Path(base path="Data Directory", name or relative path=w381) -> (appended path=w378:path)
            n149 = local write "Filenumber"(w379) -> ()
            n150 = Build Path(base path="Data Directory", name or relative path=w374) -> (appended path=w372:path)
            n151 = Concatenate Strings(w328, "\r", "Comments and Experimental Notes") -> (w350:string)
            n152 = Open/Create/Replace File(file path (use dialog)=w365, operation (0:open)=T1."create") -> (refnum out=w360:refnum<file>)  [unwired: 4 in, 2 out]
            n153 = Open/Create/Replace File(file path (use dialog)=w378, operation (0:open)=T1."create") -> ()  [unwired: 4 in, 3 out]
            n154 = Open/Create/Replace File(file path (use dialog)=w372, operation (0:open)=T1."create") -> (refnum out=w371:refnum<file>)  [unwired: 4 in, 2 out]
            n155 = Write to Text File(file (use dialog)=w360, text=w350) -> (refnum out=w359:refnum<file>)  [unwired: 2 in, 2 out]
            n156 = call-poly <vilib>:"Write To Spreadsheet File.vi"("delimiter (\\t)"=",", "format (%.3f)"="%e", "2D data"=w333, "file path (dialog if empty)"=w378) -> ()  [unwired: 4 in, 1 out]
            n157 = Close File(refnum=w359) -> ()  [unwired: 1 in, 2 out]
            n158 = Array Size(array=w333) -> ()  [unwired: 1 out]
            n159 = Index Array(array=w333, index (col)=0) -> (element=w342:dbl[])  [unwired: 1 in]
            n160 = Index Array(array=w333, index (col)=1) -> (element=w341:dbl[])  [unwired: 1 in]
            n161 = Index Array(array=w333, index (col)=2) -> (element=w340:dbl[])  [unwired: 1 in]
            n162 = Index Array(array=w333, index (col)=5) -> (element=w337:dbl[])  [unwired: 1 in]
            n163 = Index Array(array=w333, index (col)=3) -> (element=w339:dbl[])  [unwired: 1 in]
            n164 = Index Array(array=w333, index (col)=4) -> (element=w338:dbl[])  [unwired: 1 in]
            n165 = Index Array(array=w333, index (col)=6) -> (element=w336:dbl[])  [unwired: 1 in]
            n166 = Bundle(w342, w341, w340, w339, w338, w337, w336) -> ()  [unwired: 1 in, 1 out]
            n167 = Write to Binary File(file (use dialog)=w371, data=w333, 5:TRUE ("prepend array or string size? (T)")) -> (refnum out=w369:refnum<file>)  [unwired: 3 in, 2 out]
            n168 = local write "Save Indicator"(TRUE) -> ()
            n169 = local write "Save IV"(FALSE) -> ()
            n170 = Close File(refnum=w369) -> ()  [unwired: 1 in, 2 out]
          }
          frame 5 {
            n171 = property on="DATA Filename" class="Str"() -> ("Value"=w397:string)  [unwired: 2 in, 2 out]
            n172 = Number To Engineering String(2:i16 8 ("width (-)"), 4:w384) -> (0:w383:string[])  [unwired: 2 in]
            n173 = Concatenate Strings(w397, "_Decay.txt") -> (w401:string)
            n174 = Concatenate Strings(w397, "_Decay.acq") -> (w395:string)
            n175 = property on="Data Directory" class="Path"() -> ("Value"=w394:path)  [unwired: 2 in, 2 out]
            n176 = Build Path(base path=w394, name or relative path=w395) -> (appended path=w393:path)
            n177 = Build Path(base path=w394, name or relative path=w401) -> (appended path=w400:path)
            n178 = Open/Create/Replace File(file path (use dialog)=w393, operation (0:open)=T1."create") -> (refnum out=w399:refnum<file>)  [unwired: 4 in, 2 out]
            n179 = Build Array(w385, w383) -> (w390:string[][])
            n180 = Transpose 2D Array(2D array=w390) -> (transposed array=w389:string[][])
            n181 = Write to Binary File(file (use dialog)=w399, data=w389, 5:FALSE ("prepend array or string size? (T)")) -> (refnum out=w398:refnum<file>)  [unwired: 3 in, 2 out]
            n182 = call-poly <vilib>:"Write To Spreadsheet File.vi"("format (%s)"="%e", "2D data"=w389, "file path (dialog if empty)"=w400) -> ()  [unwired: 5 in, 1 out]
            n183 = Close File(refnum=w398) -> ()  [unwired: 1 in, 2 out]
          }
          frame 6 {
            (unwired) 100000
            w409 = 0.0
            w431 = 10123 items=["Finite Samples"=10178, "Continuous Samples"=10123] ("sample mode")
            w435 = T2 3 items=["no dialog", "OK message", "continue or stop message", "OK message + warnings", "continue/stop + warnings"] ("type of dialog (OK msg:1)")
            w439 = 10123 items=["Finite Samples"=10178, "Continuous Samples"=10123, "Hardware Timed Single Point"=12522] ("sample mode")
            n184 = call-poly <vilib>:"DAQmx Create Virtual Channel.vi"("maximum value"=10.0 ("maximum value 2"), "minimum value"=-10.0 ("minimum value 2"), "physical channels"=tag "Dev1/ao1" ("physical channels 2")) -> ("task out"=w441:refnum<k21>, "error out"=w440:errorcluster)  [unwired: 11 in]
            n185 = call-poly <vilib>:"DAQmx Create Virtual Channel.vi"("maximum value"=10.0 ("Maximum Value 2"), "minimum value"=-10.0 ("Minimum Value 2"), "physical channels"=tag "Dev1/ai0" ("Physical Channel 2")) -> ("task out"=w429:refnum<k21>, "error out"=w430:errorcluster)  [unwired: 11 in]
            n186 = call-poly <vilib>:"DAQmx Timing.vi"("task/channels in"=w429, "sample mode"=w431, "samples per channel"=2, "rate"=5000.0 ("Rate 2"), "error in"=w430) -> ("task out"=w425:refnum<k21>, "error out"=w424:errorcluster)  [unwired: 9 in]
            n187 = call-poly <vilib>:"DAQmx Timing.vi"("task/channels in"=w441, "sample mode"=w439, "rate"=5000, "error in"=w440) -> ("task out"=w438:refnum<k21>, "error out"=w437:errorcluster)  [unwired: 10 in]
            n188 = property class="DAQmx Timing" props=["Sample Clock:Rate"](reference=w425, error in=w424) -> (reference out=w423:refnum<k21>, error out=w422:errorcluster)  [unwired: 1 out]
            n189 = call <vilib>:"DAQmx Start Task.vi"("task/channels in"=w438, "error in"=w437) -> ("task out"=w436:refnum<k21>, "error out"=w418:errorcluster)  [unwired: 12 in]
            n190 = call "Get Terminal Name with Device Prefix.vi"("error in (no error)"=w422, "Local Terminal Name"="ai/StartTrigger" ("terminal"), "task/channels in"=w423) -> ("error out"=w406:errorcluster, "task out"=w407:refnum<k21>)  [unwired: 6 in, 1 out]
            n191 = property on="Waveform Chart" class="WFChart (strict)"("Visible"=TRUE) -> ()  [unwired: 2 in, 2 out]
            n192 = call <vilib>:"DAQmx Start Task.vi"("task/channels in"=w407, "error in"=w406) -> ("task out"=w416:refnum<k21>, "error out"=w420:errorcluster)  [unwired: 12 in]
            n193 = Initialize Array(w409, w409) -> ()  [unwired: 1 out]
            n194 = while {
              tunnel: w436 -> [w467]
              tunnel: w420 -> [w466]
              tunnel: w418 -> [w465]
              tunnel: ["Analog Ouyput 1"] -> w417
              tunnel: w416 -> [w464]
              tunnel: [w463] -> w415
              tunnel: [w462] -> w414
              tunnel: [w461] -> w412
              tunnel: [w455] -> w410
              stop <- w452 stop-if-true
              n195 = call-poly <vilib>:"DAQmx Read.vi"("task/channels in"=w464, "error in"=w466) -> ("task out"=w455:refnum<k21>, "data"=w450:dbl, "error out"=w461:errorcluster)  [unwired: 11 in]
              "Waveform Chart" <- w450
              n196 = call-poly <vilib>:"DAQmx Write.vi"("task/channels in"=w467, "data"="Analog Ouyput 1", "timeout"=0.1 ("Wirite Timeout"), "error in"=w465) -> ("task out"=w463:refnum<k21>, "error out"=w462:errorcluster)  [unwired: 9 in, 1 out]
              n197 = local read "Manual Z"() -> (w449:bool)
              n198 = local read "Sweep Bias"() -> (w453:bool)
              n199 = local read "Save IV"() -> (w451:bool)
              n200 = Build Array("Analog Ouyput 1") -> (w459:dbl[])
              n201 = Build Array(w450) -> (w458:dbl[])
              n202 = Build Array(w458, w459) -> (w457:dbl[][])
              n203 = Not(x=w449) -> (.not. x?=w454:bool)
              n204 = Transpose 2D Array(2D array=w457) -> ()  [unwired: 1 out]
              n205 = Compound Arithmetic op=OR(w451, w453, w454) -> (w452:bool)
            }
            n206 = call <vilib>:"DAQmx Clear Task.vi"("task in"=w415, "error in"=w414) -> ("error out"=w413:errorcluster)  [unwired: 13 in]
            n207 = call <vilib>:"DAQmx Clear Task.vi"("task in"=w410, "error in"=w412) -> ("error out"=w411:errorcluster)  [unwired: 13 in]
            n208 = Merge Errors(w411, w413) -> (w419:errorcluster)
            n209 = call <vilib>:"General Error Handler.vi"("type of dialog (OK msg:1)"=w435, "error in (no error)"=w419) -> ()  [unwired: 9 in, 5 out]
          }
          frame 7 {
            w471 = 0.0
            w492 = T2 3 items=["no dialog", "OK message", "continue or stop message", "OK message + warnings", "continue/stop + warnings"] ("type of dialog (OK msg:1)")
            w507 = 10123 items=["Finite Samples"=10178, "Continuous Samples"=10123] ("sample mode")
            w501 = 10123 items=["Finite Samples"=10178, "Continuous Samples"=10123] ("sample mode")
            n210 = call-poly <vilib>:"DAQmx Create Virtual Channel.vi"("maximum value"=10.0 ("maximum value 2"), "minimum value"=-10.0 ("minimum value 2"), "physical channels"=tag "Dev1/ao1" ("physical channels 2")) -> ("task out"=w508:refnum<k21>, "error out"=w509:errorcluster)  [unwired: 11 in]
            n211 = call-poly <vilib>:"DAQmx Create Virtual Channel.vi"("maximum value"=10.0 ("Maximum Value 2"), "minimum value"=-10.0 ("Minimum Value 2"), "physical channels"=tag "Dev1/ai0" ("Physical Channel 2")) -> ("task out"=w503:refnum<k21>, "error out"=w502:errorcluster)  [unwired: 11 in]
            n212 = call-poly <vilib>:"DAQmx Timing.vi"("task/channels in"=w508, "sample mode"=w507, "rate"=10000.0 ("rate 2"), "error in"=w509) -> ("task out"=w516:refnum<k21>, "error out"=w517:errorcluster)  [unwired: 10 in]
            n213 = call-poly <vilib>:"DAQmx Timing.vi"("task/channels in"=w503, "sample mode"=w501, "rate"=10000.0 ("Rate 2"), "error in"=w502) -> ("task out"=w519:refnum<k21>, "error out"=w520:errorcluster)  [unwired: 10 in]
            n214 = property class="DAQmx Timing" props=["Sample Clock:Rate"](reference=w516, error in=w517) -> (reference out=w515:refnum<k21>, error out=w518:errorcluster)  [unwired: 1 out]
            n215 = property class="DAQmx Timing" props=["Sample Clock:Rate"](reference=w519, error in=w520) -> (reference out=w521:refnum<k21>, error out=w522:errorcluster)  [unwired: 1 out]
            n216 = call "Get Terminal Name with Device Prefix.vi"("error in (no error)"=w522, "Local Terminal Name"="ai/StartTrigger" ("terminal"), "task/channels in"=w521) -> ("error out"=w490:errorcluster, "Terminal Name with Device Prefix"=w514:tag, "task out"=w488:refnum<k21>)  [unwired: 6 in]
            n217 = call-poly <vilib>:"DAQmx Trigger.vi"("task/channels in"=w515, "source"=w514, "error in"=w518) -> ("task out"=w483:refnum<k21>, "error out"=w480:errorcluster)  [unwired: 11 in]
            n218 = Initialize Array(0.0, "Step Length") -> (w486:dbl[])
            n219 = call <vilib>:"DAQmx Start Task.vi"("task/channels in"=w488, "error in"=w490) -> ("task out"=w487:refnum<k21>, "error out"=w489:errorcluster)  [unwired: 12 in]
            n220 = call <vilib>:"DAQmx Start Task.vi"("task/channels in"=w483, "error in"=w480) -> ("task out"=w482:refnum<k21>, "error out"=w481:errorcluster)  [unwired: 12 in]
            n221 = Initialize Array(w471, w471) -> (w470:dbl[])
            n222 = while {
              tunnel: w487 -> [w543]
              tunnel: w489 -> [w542]
              tunnel: w482 -> [w541]
              tunnel: w481 -> [w540]
              tunnel: [w539] -> w498
              tunnel: [w538] -> w497
              tunnel: [w537] -> w495
              tunnel: [w536] -> w493
              shift-right: [w534] -> _
              shift-left: w486 -> [w535]
              tunnel: w478 -> [w532]
              shift-right: [w531] -> _
              shift-left: 1 -> [w530]
              shift-right: [w529] -> w474
              shift-left: w479 -> [w533]
              shift-right: [w527] -> w473
              shift-left: w470 -> [w528]
              shift-right: [w525] -> w472
              shift-left: w470 -> [w526]
              tunnel: [w523] -> w469
              stop <- w523 stop-if-true
              n223 = stacked-sequence {
                seq-local: [w545 _] -> [_ w585]
                tunnel: w543 -> [w576 _]
                tunnel: w542 -> [w575 _]
                tunnel: w541 -> [_ w593]
                tunnel: w540 -> [_ w592]
                tunnel: [w573 _] -> w539
                tunnel: [w574 _] -> w538
                tunnel: [_ w590] -> w537
                tunnel: [_ w591] -> w536
                tunnel: w535 -> [w570 w577]
                tunnel: [w553 _] -> w534
                tunnel: [w546 _] -> w523
                tunnel: w533 -> [_ w589]
                tunnel: w532 -> [_ w588]
                tunnel: [_ w587] -> w531
                tunnel: w530 -> [w562 w586]
                tunnel: "Ramp Rate" -> [_ w584]
                tunnel: [_ w582] -> _
                tunnel: [_ w582] -> w529
                tunnel: w528 -> [_ w581]
                tunnel: [_ w580] -> w527
                tunnel: w526 -> [_ w579]
                tunnel: [_ w578] -> w525
                frame #0 {
                  n224 = call-poly <vilib>:"DAQmx Read.vi"("task/channels in"=w576, "error in"=w575) -> ("task out"=w573:refnum<k21>, "data"=w544:dbl, "error out"=w574:errorcluster)  [unwired: 11 in]
                  n225 = Absolute Value(x=w544) -> (abs(x)=w545:dbl)
                  n226 = Insert Into Array(array=w570, index=0, new element=w545) -> (w571:dbl[])
                  n227 = local write "Waveform Chart"(w545) -> ()
                  n228 = Delete From Array(array=w571, length=1) -> (array with subset deleted=w553:dbl[])  [unwired: 1 in, 1 out]
                  n229 = Array Size(array=w553) -> (size(s)=w563:i32)
                  n230 = Decrement(x=w563) -> (x-1=w554:i32)
                  n231 = Index Array(array=w553, index=w554) -> (element=w556:dbl)
                  "element" <- w556
                  n232 = Index Array(array=w553, index=0) -> (element=w558:dbl)
                  n233 = Less?(x=w553, y="Step Max") -> (x < y?=w568:bool[])
                  n234 = Greater?(x=w553, y="Step Min") -> (0:w567:bool[])
                  n235 = Greater?(x="Step Min", y=w556) -> ()  [unwired: 1 out]
                  n236 = And Array Elements(Boolean array=w568) -> (logical AND=w552:bool)
                  n237 = And Array Elements(Boolean array=w567) -> (logical AND=w551:bool)
                  n238 = Less?(x="Step Max", y=w558) -> ()  [unwired: 1 out]
                  n239 = local read "Tapping"() -> (w548:bool)
                  n240 = And(x=w552, y=w551) -> (x .and. y?=w566:bool)
                  n241 = Equal?(x=w562, y=1) -> (x = y?=w560:bool)
                  n242 = Equal?(x=w562, y=2) -> (x = y?=w559:bool)
                  n243 = Or(x=w560, y=w559) -> (x .or. y?=w550:bool)
                  n244 = Not(x=w548) -> (.not. x?=w547:bool)
                  n245 = Compound Arithmetic op=AND(w566, w550) -> (w549:bool)
                  "Tapping Stop" <- w549
                  n246 = Or(x=w549, y=w547) -> (x .or. y?=w546:bool)
                }
                frame #1 {
                  n247 = case shown="1, Default" w586 {
                    tunnel: [w601 w624 w645 w671] -> w582
                    tunnel: w589 -> [w614 w626 w656 w668]
                    tunnel: [w609 w625 w650 w667] -> w587
                    tunnel: w585 -> [w600 _ w655 _]
                    tunnel: w584 -> [w615 w629 w657 w666]
                    tunnel: w581 -> [w605 w623 w644 _]
                    tunnel: [w607 w623 w644 w664] -> w580
                    tunnel: w579 -> [w599 w622 w643 _]
                    tunnel: [w606 w622 w643 w664] -> w578
                    tunnel: w577 -> [w598 _ _ _]
                    frame 1, Default {
                      w603 = -10
                      # "Breaking the contact"
                      n248 = Divide(x=w615, y=15.13) -> (x/y=w619:dbl)
                      n249 = Array Subset(array=w598, index=0, length=10) -> (w595:dbl[])
                      n250 = Divide(x=20, y=32768) -> (x/y=w616:dbl)
                      n251 = call-poly <vilib>:"Mean.vi"("X"=w595) -> ("mean"=w594:dbl)  [unwired: 1 out]
                      "mean" <- w594
                      n252 = Multiply(x=w616, y=w619) -> (x*y=w621:dbl)
                      n253 = Subtract(x=w614, y=w621) -> (x-y=w602:dbl)
                      n254 = Less?(x=w594, y="Min Current") -> (x < y?=w612:bool)
                      n255 = Select(t=2, s=w612, f=1) -> (s? t:f=w609:i32)
                      n256 = Build Array (concatenate)(w602, w605) -> (w607:dbl[])
                      n257 = Build Array (concatenate)(w600, w599) -> (w606:dbl[])
                      n258 = Less?(x=w602, y=w603) -> (x < y?=w604:bool)
                      n259 = local write "Contact Cycles"(0) -> ()
                      n260 = Select(t=w603, s=w604, f=w602) -> (s? t:f=w601:dbl)
                    }
                    frame 2 {
                      w641 = 10
                      # "Break contact cycles after current = 0"
                      n261 = Divide(x=w629, y=15.13) -> (x/y=w637:dbl)
                      n262 = local read "Contact Cycles"() -> (w628:i32)
                      n263 = Divide(x=20, y=32768) -> (x/y=w630:dbl)
                      n264 = Multiply(x=w630, y=w637) -> (x*y=w639:dbl)
                      n265 = Subtract(x=w626, y=w639) -> (x-y=w631:dbl)
                      n266 = Increment(x=w628) -> (x+1=w627:i32)
                      n267 = Less?(x=w631, y=w641) -> (x < y?=w640:bool)
                      n268 = Select(t=w631, s=w640, f=w641) -> (s? t:f=w624:dbl)
                      n269 = Less Or Equal?(x="Break Contact", y=w627) -> (x <= y?=w634:bool)
                      n270 = local write "Contact Cycles"(w627) -> ()
                      n271 = Select(t=3, s=w634, f=2) -> (s? t:f=w625:i32)
                    }
                    frame 3 {
                      w648 = 10
                      # "Making contact"
                      n272 = Divide(x=w657, y=15.13) -> (x/y=w661:dbl)
                      n273 = Divide(x=20, y=32768) -> (x/y=w658:dbl)
                      n274 = Multiply(x=w658, y=w661) -> (x*y=w663:dbl)
                      n275 = Add(x=w656, y=w663) -> (x+y=w646:dbl)
                      n276 = Greater?(x=w655, y="Max Current") -> (0:w653:bool)
                      n277 = Select(t=4, s=w653, f=3) -> (s? t:f=w650:i32)
                      n278 = local write "Contact Cycles"(0) -> ()
                      n279 = Less?(x=w646, y=w648) -> (x < y?=w647:bool)
                      n280 = Select(t=w646, s=w647, f=w648) -> (s? t:f=w645:dbl)
                    }
                    frame 4 {
                      w665 = 0.0
                      w683 = 10
                      # "Make contact cycles after current saturation"
                      n281 = Divide(x=w666, y=15.13) -> (x/y=w679:dbl)
                      n282 = local read "Contact Cycles"() -> (w673:i32)
                      n283 = Divide(x=20, y=32768) -> (x/y=w669:dbl)
                      n284 = Multiply(x=w669, y=w679) -> (x*y=w681:dbl)
                      n285 = Add(x=w668, y=w681) -> (x+y=w670:dbl)
                      n286 = Increment(x=w673) -> (x+1=w672:i32)
                      n287 = Less?(x=w670, y=w683) -> (x < y?=w682:bool)
                      n288 = Select(t=w670, s=w682, f=w683) -> (s? t:f=w671:dbl)
                      n289 = Less Or Equal?(x="Make Contact", y=w672) -> (x <= y?=w676:bool)
                      n290 = local write "Contact Cycles"(w672) -> ()
                      n291 = Initialize Array(w665, w665) -> (w664:dbl[])
                      n292 = Select(t=1, s=w676, f=4) -> (s? t:f=w667:i32)
                    }
                  }
                  n293 = local write "Analog Ouyput 1"(w582) -> ()
                  n294 = Build Array(w588, w582) -> ()  [unwired: 1 out]
                  n295 = call-poly <vilib>:"DAQmx Write.vi"("task/channels in"=w593, "auto start"=TRUE, "data"=w582, "error in"=w592) -> ("task out"=w591:refnum<k21>, "error out"=w590:errorcluster)  [unwired: 9 in, 1 out]
                }
              }
              "Case" <- w531
            }
            n296 = call <vilib>:"DAQmx Clear Task.vi"("task in"=w493, "error in"=w495) -> ("error out"=w494:errorcluster)  [unwired: 13 in]
            n297 = Not(x=w469) -> (.not. x?=w468:bool)
            n298 = call <vilib>:"DAQmx Clear Task.vi"("task in"=w498, "error in"=w497) -> ("error out"=w496:errorcluster)  [unwired: 13 in]
            n299 = local write "Tapping"(w468) -> ()
            n300 = Merge Errors(w496, w494) -> (w491:errorcluster)
            n301 = call <vilib>:"General Error Handler.vi"("type of dialog (OK msg:1)"=w492, "error in (no error)"=w491) -> ()  [unwired: 9 in, 5 out]
          }
          frame 8 {
            w690 = 0.0
            w704 = T2 3 items=["no dialog", "OK message", "continue or stop message", "OK message + warnings", "continue/stop + warnings"] ("type of dialog (OK msg:1)")
            w717 = 10123 items=["Finite Samples"=10178, "Continuous Samples"=10123] ("sample mode")
            w711 = 10123 items=["Finite Samples"=10178, "Continuous Samples"=10123] ("sample mode")
            n302 = call-poly <vilib>:"DAQmx Create Virtual Channel.vi"("maximum value"=10.0 ("maximum value 2"), "minimum value"=-10.0 ("minimum value 2"), "physical channels"=tag "Dev1/ao0:1" ("physical channels 2")) -> ("task out"=w718:refnum<k21>, "error out"=w719:errorcluster)  [unwired: 11 in]
            n303 = call-poly <vilib>:"DAQmx Create Virtual Channel.vi"("maximum value"=10.0 ("Maximum Value 2"), "minimum value"=-10.0 ("Minimum Value 2"), "physical channels"=tag "Dev1/ai0" ("Physical Channel 2")) -> ("task out"=w713:refnum<k21>, "error out"=w712:errorcluster)  [unwired: 11 in]
            n304 = call-poly <vilib>:"DAQmx Timing.vi"("task/channels in"=w718, "sample mode"=w717, "rate"=10000.0 ("rate 2"), "error in"=w719) -> ("task out"=w726:refnum<k21>, "error out"=w727:errorcluster)  [unwired: 10 in]
            n305 = call-poly <vilib>:"DAQmx Timing.vi"("task/channels in"=w713, "sample mode"=w711, "rate"=10000.0 ("Rate 2"), "error in"=w712) -> ("task out"=w729:refnum<k21>, "error out"=w730:errorcluster)  [unwired: 10 in]
            n306 = property class="DAQmx Timing" props=["Sample Clock:Rate"](reference=w726, error in=w727) -> (reference out=w725:refnum<k21>, error out=w728:errorcluster)  [unwired: 1 out]
            n307 = property class="DAQmx Timing" props=["Sample Clock:Rate"](reference=w729, error in=w730) -> (reference out=w731:refnum<k21>, error out=w732:errorcluster)  [unwired: 1 out]
            n308 = call "Get Terminal Name with Device Prefix.vi"("error in (no error)"=w732, "Local Terminal Name"="ai/StartTrigger" ("terminal"), "task/channels in"=w731) -> ("error out"=w702:errorcluster, "Terminal Name with Device Prefix"=w724:tag, "task out"=w700:refnum<k21>)  [unwired: 6 in]
            n309 = call-poly <vilib>:"DAQmx Trigger.vi"("task/channels in"=w725, "source"=w724, "error in"=w728) -> ("task out"=w698:refnum<k21>, "error out"=w695:errorcluster)  [unwired: 11 in]
            n310 = call <vilib>:"DAQmx Start Task.vi"("task/channels in"=w700, "error in"=w702) -> ("task out"=w699:refnum<k21>, "error out"=w701:errorcluster)  [unwired: 12 in]
            n311 = call <vilib>:"DAQmx Start Task.vi"("task/channels in"=w698, "error in"=w695) -> ("task out"=w697:refnum<k21>, "error out"=w696:errorcluster)  [unwired: 12 in]
            n312 = Initialize Array(w690, w690) -> ()  [unwired: 1 out]
            n313 = while {
              tunnel: w699 -> [w767]
              tunnel: w701 -> [w766]
              tunnel: w697 -> [w756]
              tunnel: w696 -> [w755]
              tunnel: [w765] -> w708
              tunnel: [w764] -> w707
              shift-right: [w741] -> w691
              shift-left: w694 -> [w746]
              tunnel: [w754] -> w689
              tunnel: [w753] -> w688
              tunnel: w685 -> [w737]
              i -> [w752]
              stop <- w742 stop-if-true
              w750 = 5e-05
              n314 = Absolute Value(x="Setpoint") -> (abs(x)=w733:dbl)
              n315 = call-poly <vilib>:"DAQmx Read.vi"("task/channels in"=w767, "error in"=w766) -> ("task out"=w765:refnum<k21>, "data"=w736:dbl, "error out"=w764:errorcluster)  [unwired: 11 in]
              n316 = Absolute Value(x=w736) -> (abs(x)=w735:dbl)
              n317 = local read "Bias Offset Correct"() -> (w738:dbl)
              n318 = Bundle("Proportional Gain"="Proportional Gain", "Integral Gain"="Integral Gain", "Differential Gain"="Differential Gain") -> (w757:T3)  [unwired: 1 in]
              n319 = local write "Waveform Chart"(w736) -> ()
              n320 = Bundle(10, -10) -> (w761:cluster{i32, i32})  [unwired: 1 in]
              n321 = call-poly "PID.vi"("output range"=w761, "dt (s)"=w750, "PID gains"=w757, "process variable"=w735, "setpoint"=w733) -> ("output"=w749:dbl)  [unwired: 5 in, 1 out]
              n322 = Add(x=w737, y=w738) -> (x+y=w739:dbl)
              n323 = Less?(x=w752, y=1000) -> (x < y?=w747:bool)
              n324 = call-poly "PID Output Rate Limiter.vi"("reinitialize? (F)"=w747, "dt (s)"=w750, "output rate (EGU/min)"="Piezo Delta rate", "initial output"=w746, "input (controller output)"=w749) -> ("output"=w741:dbl)  [unwired: 3 in, 1 out]
              n325 = local write "Analog Ouyput 1"(w741) -> ()
              n326 = Build Array(w739, w741) -> (w740:dbl[])
              n327 = local read "Sweep Bias"() -> (w745:bool)
              n328 = local read "PID"() -> (w743:bool)
              n329 = call-poly <vilib>:"DAQmx Write.vi"("task/channels in"=w756, "data"=w740, "error in"=w755) -> ("task out"=w754:refnum<k21>, "error out"=w753:errorcluster)  [unwired: 10 in, 1 out]
              n330 = Not(x=w743) -> (.not. x?=w744:bool)
              n331 = Compound Arithmetic op=OR(w745, w744) -> (w742:bool)
            }
            n332 = call <vilib>:"DAQmx Clear Task.vi"("task in"=w689, "error in"=w688) -> ("error out"=w705:errorcluster)  [unwired: 13 in]
            n333 = call <vilib>:"DAQmx Clear Task.vi"("task in"=w708, "error in"=w707) -> ("error out"=w706:errorcluster)  [unwired: 13 in]
            n334 = Merge Errors(w706, w705) -> (w703:errorcluster)
            n335 = call <vilib>:"General Error Handler.vi"("type of dialog (OK msg:1)"=w704, "error in (no error)"=w703) -> ()  [unwired: 9 in, 5 out]
          }
        }
      }
    }
  }
